vi "Main 2.0.vi"() -> ()   [LabVIEW 2019]
uses:
  Controls/Tab Button.ctl
  Controls/Main-state.ctl
  Controls/FGV States.ctl
  Controls/eFGV States.ctl
  <vilib>/Utility/miscctls.llb/LVRectTypeDef.ctl
  Controls/UDP - Command.ctl
  Controls/UDP - Event.ctl
  Controls/UDP - Status.ctl
  Controls/Global - Data UDP.vi
  <vilib>/httpClient/POSTBuffer.vi
  Controls/Global - IP Address.vi
  Controls/Global - Handle.vi
  Controls/Global - Handle V1.vi
  Controls/Global - Device.vi
  Controls/Global - Done.vi
  Controls/Global - Comport.vi
  Controls/Global - Unit.vi
  Controls/Global - ADC.vi
  Controls/Global - PID.vi
  Controls/Global - System.vi
  Controls/Global - Test.vi
  Controls/Global - Channel.vi
  <vilib>/httpClient/LabVIEWHTTPClient.lvlib
panel:
  out "error out":errorcluster
  out "Close Panel":T1
  in  "View 2":enum16{""}(ring) caption="Enum 3"
  in  "View":enum16{"VIEW", "Explorer", "Event Logs"}(ring) caption="Enum 3"
  in  "Instrument & Controls":T2(ring) caption="Enum 3"
  in  "Maintain Record":T3(ring) caption="Enum 3"
  in  "File":T4(ring) caption="Enum 3"
  in  "Path":path
  in  "Exit":bool
  in  "Data-Saturation":bool
  in  "Test Run1":bool
  in  "Next":bool
  in  "Previous":bool
  in  "Tab Array":T5
  in  "EventSwitch":bool
  out "Event":string caption="Event ^"
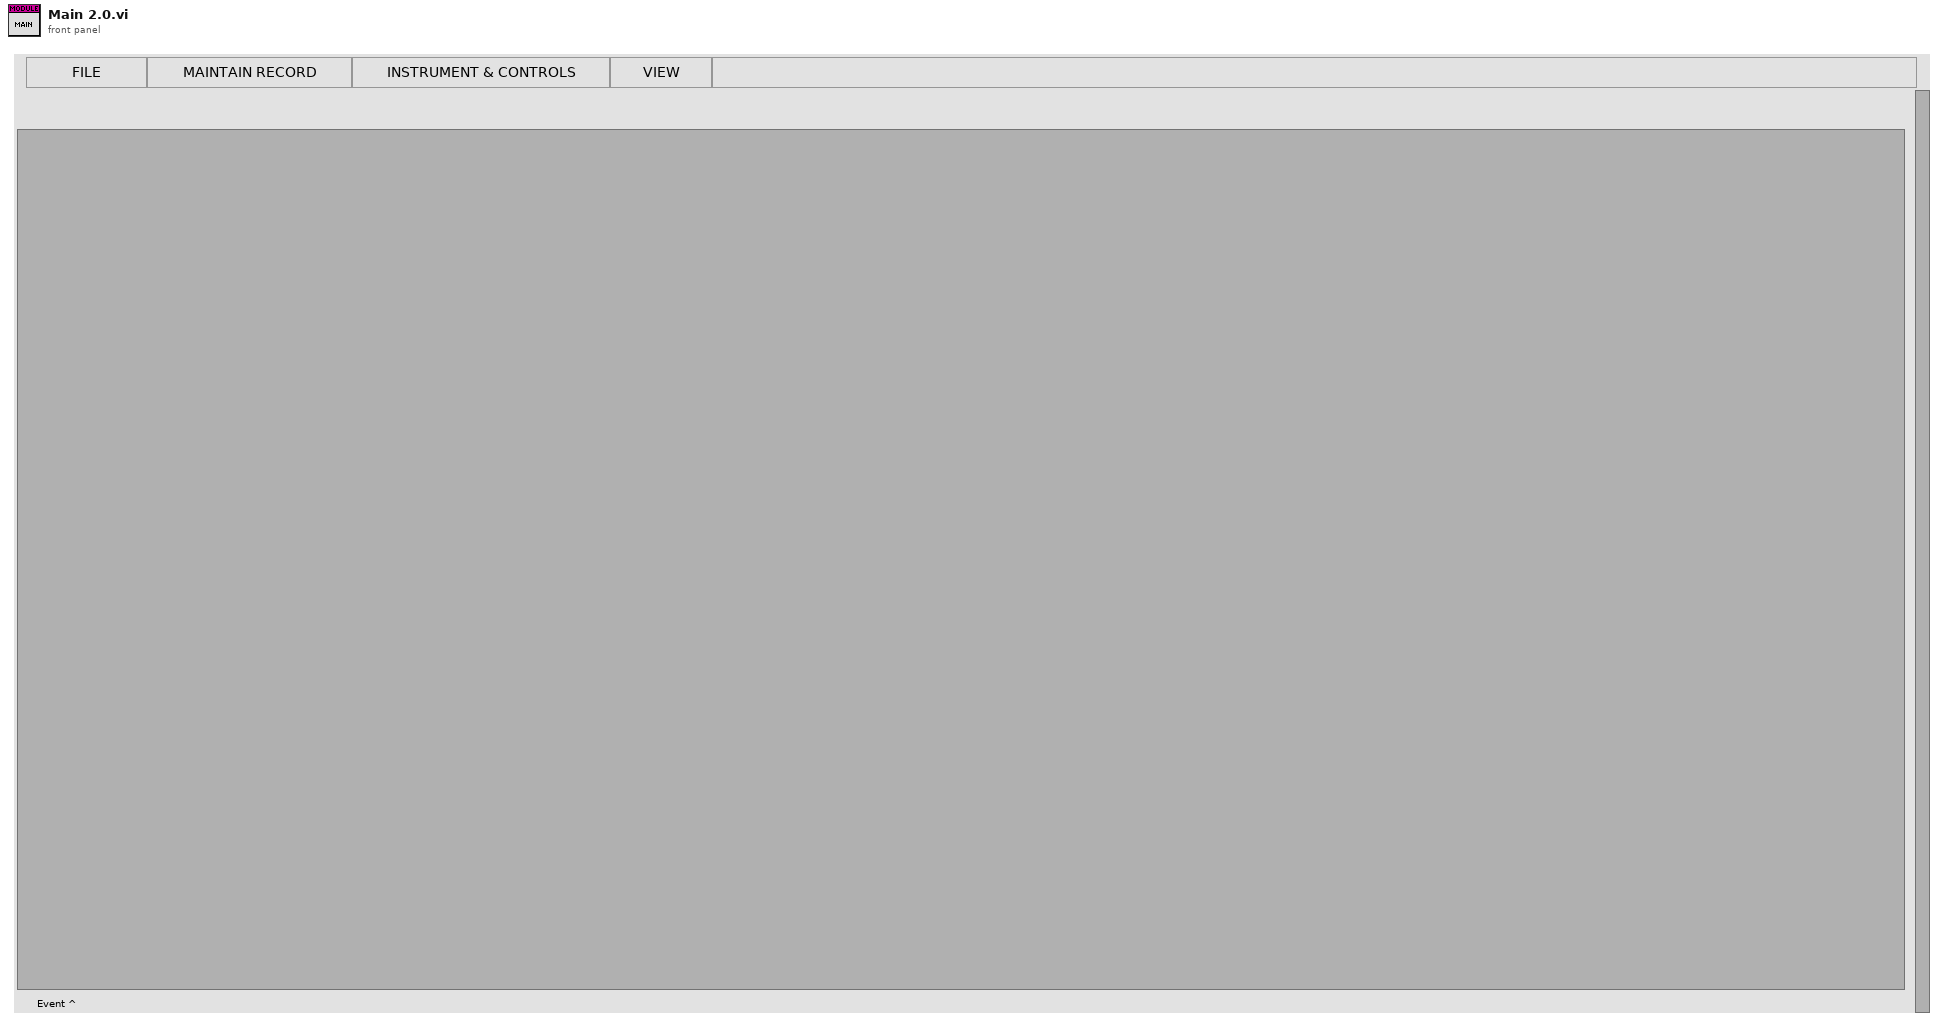
[diagram p1: front panel]
types:
  T1 = cluster{"String":string, "Cancel Button":bool, "OK Button":bool, "Bg":bool, "RunTest":refnum<vi>, "fileid":string, "Stop":bool, "Run":bool, "Status":string}
  T2 = enum16{"INSTRUMENT & CONTROLS", "Machines", "Stations", "Manual Control"}
  T3 = enum16{"MAINTAIN RECORD", "Test Plan", "Job Record"}
  T4 = enum16{"FILE", "New Test", "Export Data", "Activate License", "Emergency Stop"}
  T5 = typedef "Tab Button.ctl" = cluster{"String":string, "Cancel Button":bool, "OK Button":bool, "Bg":bool, "RunTest":refnum<vi>, "fileid":string, "Stop":bool, "Run":bool, "Status":string}[]
  T6 = enum32{"Invalid", "Standard", "Closed", "Hidden", "Minimized", "Maximized"}
  T7 = typedef "FGV States.ctl" = enum16{"Read", "Write"}
  T8 = typedef "Main-state.ctl" = enum16{"Init", "Run modules", "Idle", "Change page", "Manual Control", "NewTest", "sidepanel", "Event", "Emergency", "Exit"}
  T9 = enum32{"invalid app kind", "Development System", "Run Time System", "Student Edition", "Embedded LabVIEW", "Evaluation", "Custom"}
  T10 = cluster{"Module Ref":refnum<vi>[], "Side Name":string, "pin":bool, "FileId":string}
  T11 = typedef "eFGV States.ctl" = enum16{"Init", "Read", "Write", "Exit"}
  T12 = enum16{"New Test", "Test Plan", "Job Record", "Instrument", "Machine", "Station", "Machine Control"}
  T13 = typedef "LVRectTypeDef.ctl" = cluster{"Left":i16, "Top":i16, "Right":i16, "Bottom":i16}
  T14 = typedef "UDP - Command.ctl" = enum16{"Stop", "Jog Up", "Jog Down", "Ramp Up", "Ramp Down", "PID Target", "PID Ramp", "Disp Run", "Read Ch Data", "Zero Channel", "Zero Disp", "Read Sensor", "Write Sensor", "Read ADC", "Write ADC", "Read PID", "Write PID", "Read Test", "Write Test", "Read System", "Write System", "Read Datalog", "Read Datalog Sensor"}
  T15 = enum16{"open", "replace", "create", "open or create", "replace or create", "replace or create with confirmation"}
  T16 = cluster{"String":string, "Cancel Button":bool, "OK Button":bool, "Bg":bool, "RunTest":refnum<vi>, "fileid":string, "Stop":bool, "Run":bool, "Status":string}[]
  T17 = typedef "LabVIEWHTTPClient.lvlib/ClientHandle.ctl" = refnum<k1>
  T18 = cluster{"IP Address":string, "port":string, "UDP ref":refnum<k16>}[]
  T19 = typedef "UDP - Event.ctl" = u16
  T20 = typedef "UDP - Status.ctl" = u16
  T21 = cluster{"Channels":cluster{"Ch1":sgl, "Ch2":sgl, "Ch3":sgl, "Ch4":sgl, "Ch5":sgl, "Ch6":sgl, "Ch7":sgl, "Ch8":sgl, "Ch9":sgl, "Ch10":sgl, "Ch11":sgl, "Ch12":sgl, "Ch13":sgl, "Ch14":sgl, "Ch15":sgl, "Ch16":sgl}, "Event":T19, "Status":T20, string}[]
  T22 = cluster{"Ch1":sgl, "Ch2":sgl, "Ch3":sgl, "Ch4":sgl, "Ch5":sgl, "Ch6":sgl, "Ch7":sgl, "Ch8":sgl, "Ch9":sgl, "Ch10":sgl, "Ch11":sgl, "Ch12":sgl, "Ch13":sgl, "Ch14":sgl, "Ch15":sgl, "Ch16":sgl}
  T23 = cluster{"Target Load":sgl, "Target Disp":sgl, "Rate":sgl, "Speed":sgl}[]
  T24 = cluster{"Out Type":u8, "Inverse":u8, "Monitor":u8, "Reserve":u8, "ACC Time":u32, "Pulse Rev":u32, "Stroke":u32, "Auto Off":u32, "Gear Ratio":sgl, "Pitch":sgl, "Max Speed":u32, "Jog Speed":u32, "Disp Coff":sgl, "Max Load":u32}[]
  T25 = cluster{"SP":sgl, "PV":sgl, "kP":sgl, "kI":sgl, "kD":sgl, "FF":sgl, "Err Band":sgl, "Max":i32, "Min":i32, "Ts":u32, "Out":i32, "Mode":u8}[]
  T26 = cluster{"Active Ch":u8[], "Filter Type":u8, "Post Filter":u8[], "Gain":u8[], "FS":u16, "IntOC":u8, "IntFC":u8, "SysOC":u8, "Cofficient":dbl[], "K":dbl[], "Max":i32}[]
  T27 = cluster{"Name":string[], "Unit":string[], "Decimal Point":u8[], "Ch Log":u8[], "H Alarm":u8[], "L Alarm":u8[], "H Limit":sgl[], "L Limit":sgl[], "Filter":u8[], "Gain":u8[], "Calib Type":u32[]}[]
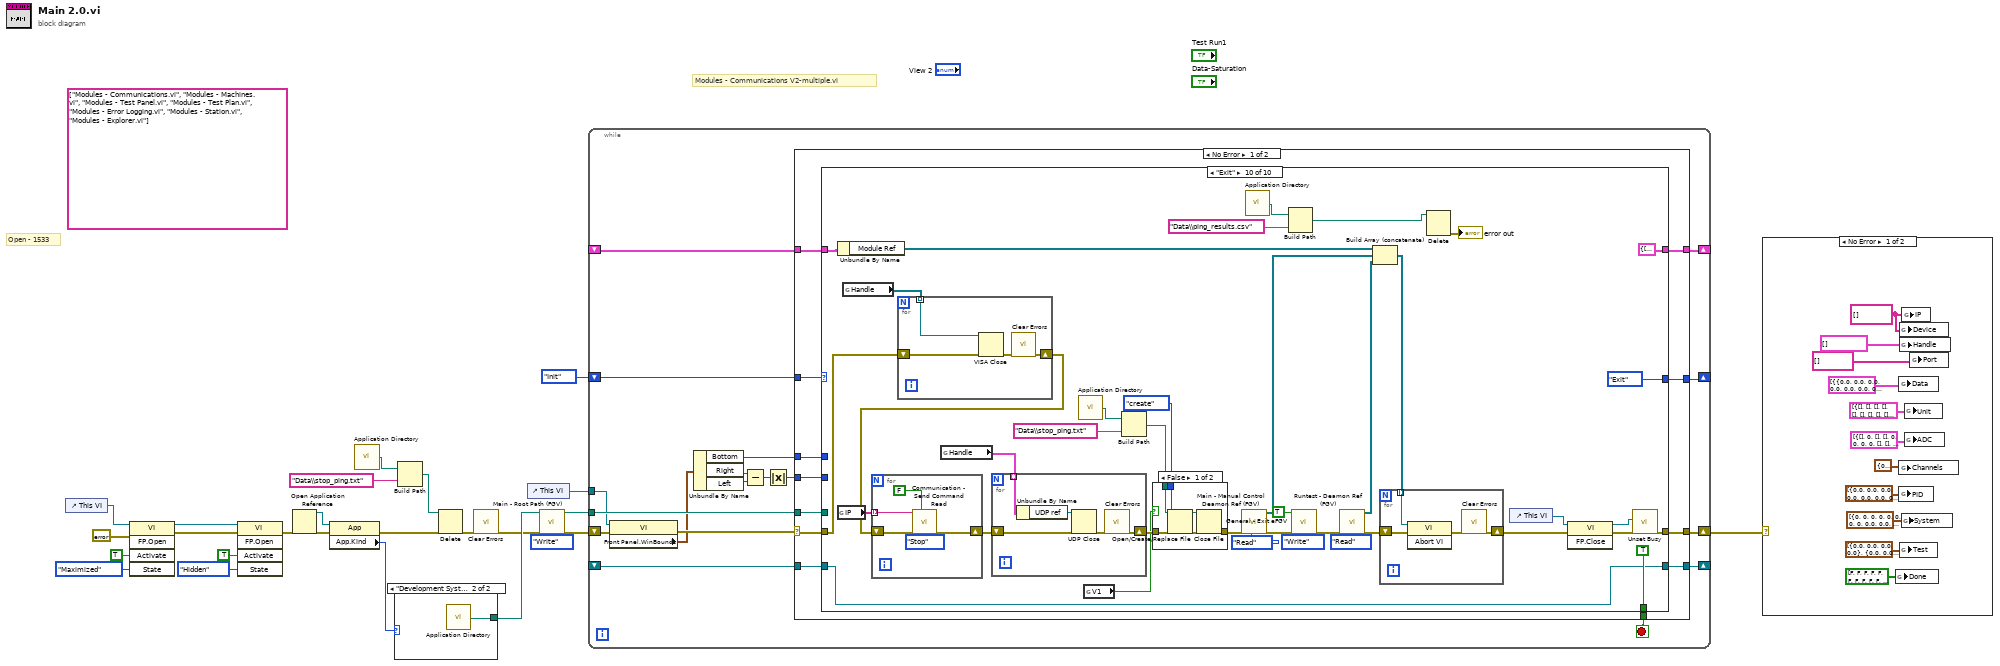
[diagram p0: block diagram]
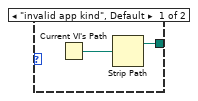
[diagram p2: hidden frame]
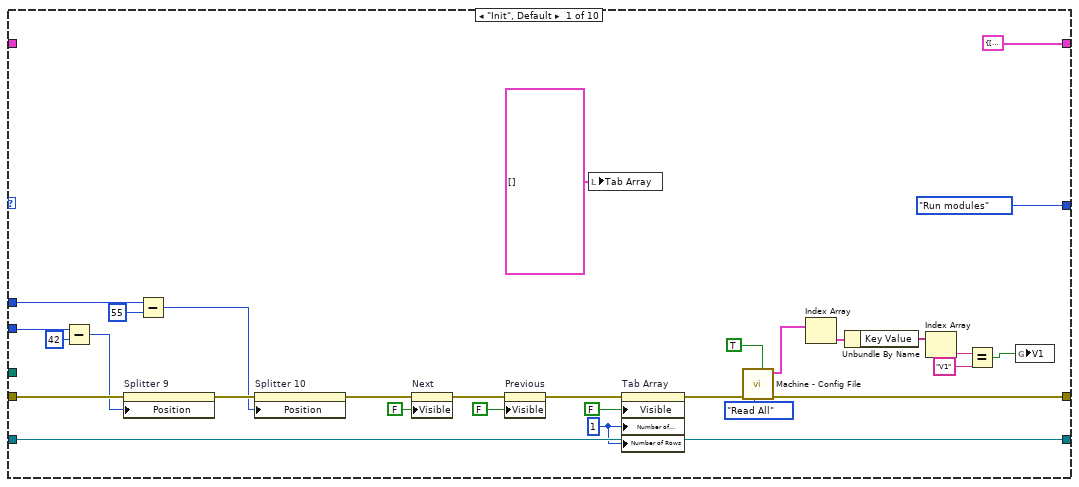
[diagram p3: hidden frame]
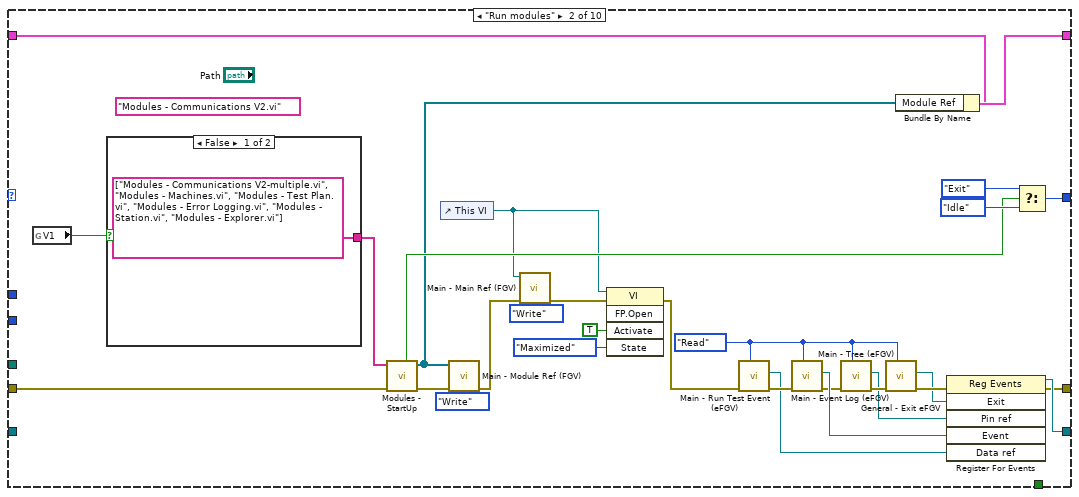
[diagram p4: hidden frame]
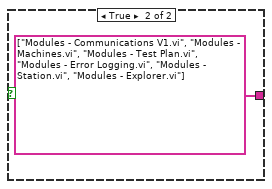
[diagram p5: hidden frame]
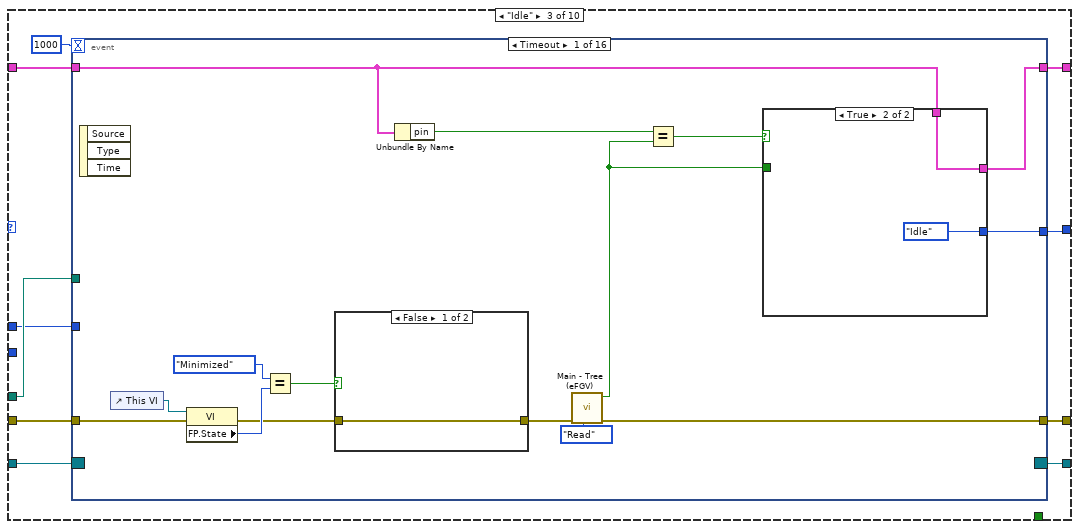
[diagram p6: hidden frame]
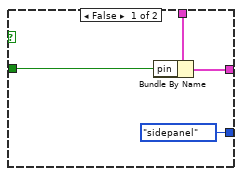
[diagram p7: hidden frame]
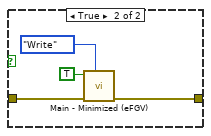
[diagram p8: hidden frame]
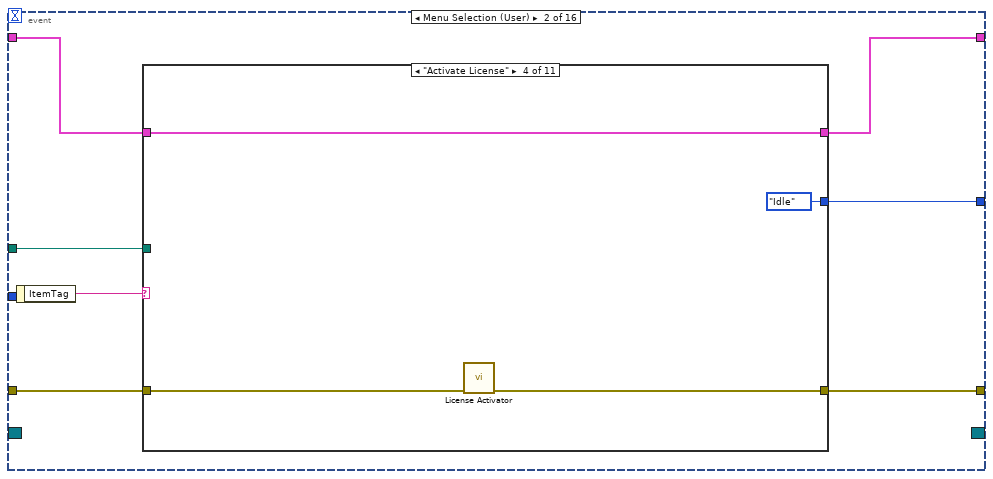
[diagram p9: hidden frame]
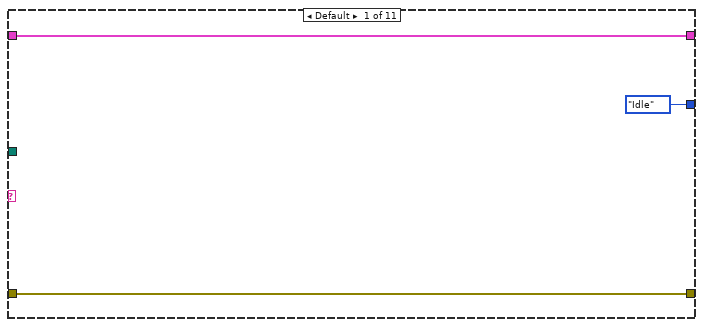
[diagram p10: hidden frame]
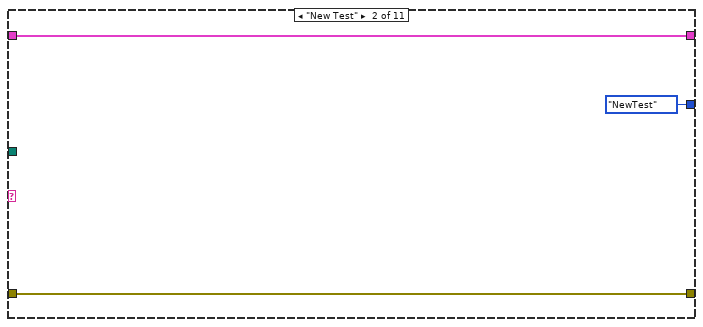
[diagram p11: hidden frame]
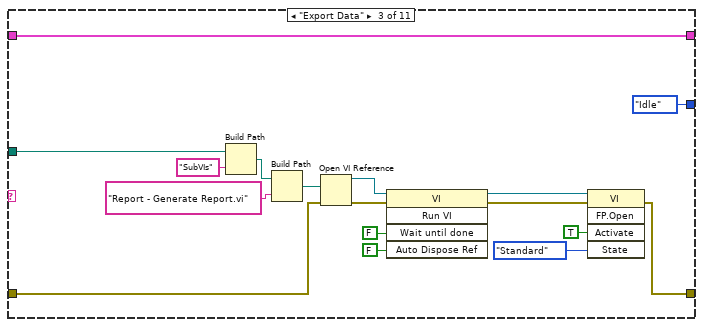
[diagram p12: hidden frame]
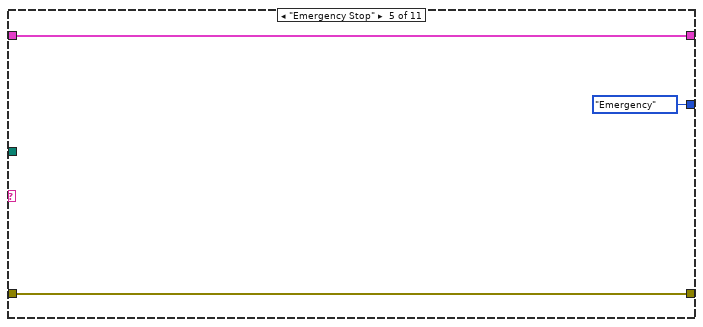
[diagram p13: hidden frame]
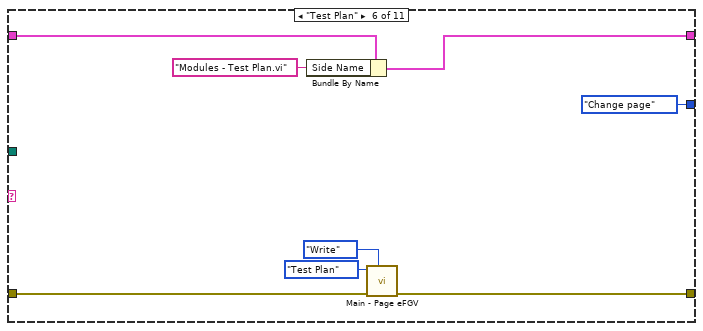
[diagram p14: hidden frame]
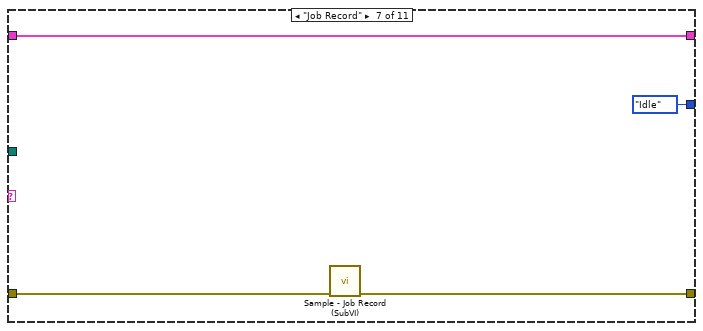
[diagram p15: hidden frame]
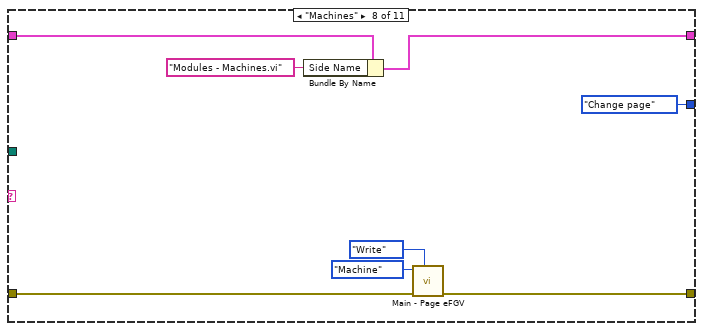
[diagram p16: hidden frame]
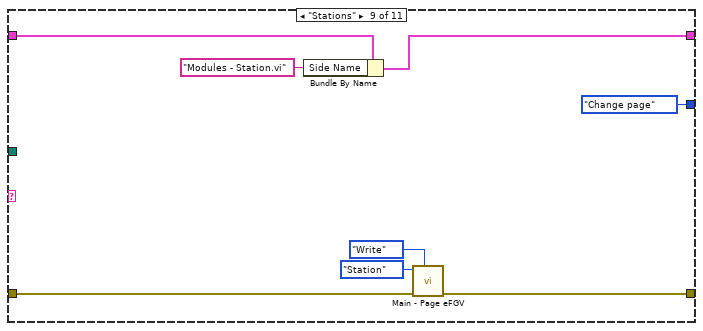
[diagram p17: hidden frame]
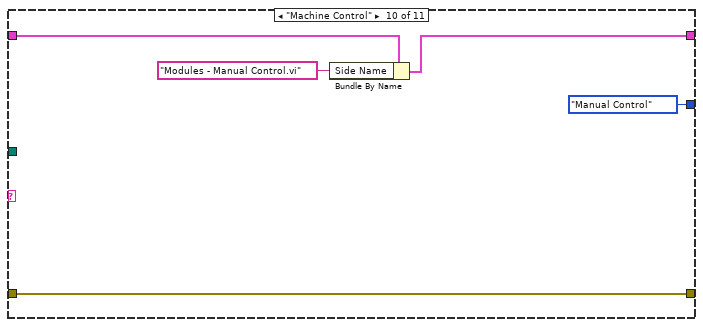
[diagram p18: hidden frame]
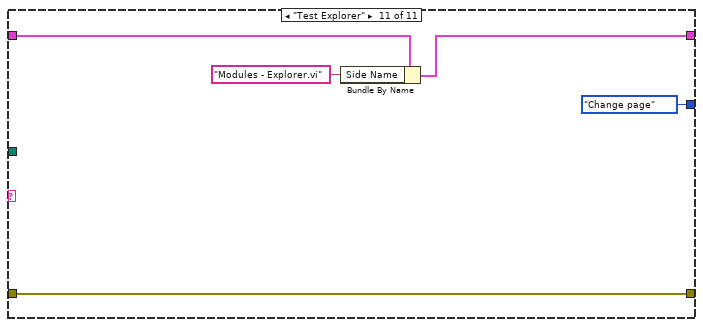
[diagram p19: hidden frame]
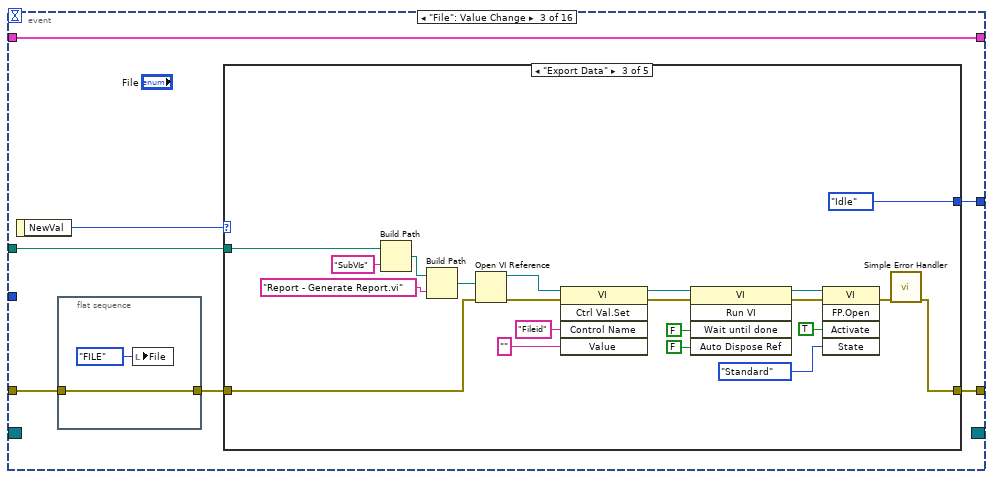
[diagram p20: hidden frame]
diagram:
  (unwired) string[] ["Modules - Communications.vi", "Modules - Machines.vi", "Modules - Test Panel.vi", "Modules - Test Plan.vi", "Modules - Error Logging.vi", "Modules - Station.vi", "Modules - Explorer.vi"]
  # "Modules - Communications V2-multiple.vi"
  # "Open - 1533"
  n1 = control-ref of="This VI"() -> (w16:refnum<vi>)
  n2 = invoke class="VI" method="FP.Open"(reference=w16, error in=errorcluster {"status"=FALSE, "code"=0, "source"=""} ("error in (no error)"), "Activate"=TRUE ("Activate?"), "State"=T6."Maximized") -> (reference out=w7:refnum<vi>, error out=w9:errorcluster)  [unwired: 1 in, 3 out]
  n3 = invoke class="VI" method="FP.Open"(reference=w7, error in=w9, "Activate"=TRUE ("Activate?"), "State"=T6."Hidden") -> (error out=w8:errorcluster)  [unwired: 1 in, 4 out]
  n4 = Open Application Reference(8:w8) -> (0:w15:errorcluster, 3:w14:refnum<vi>)  [unwired: 3 in]
  n5 = property class="App"(reference=w14, error in=w15) -> (error out=w3:errorcluster, "App.Kind"=w13:T9)  [unwired: 1 out]
  n6 = call <vilib>:"Application Directory.vi"() -> ("Application Directory"=w6:path)
  n7 = case shown="\"Development System\"" w13 {
    tunnel: [w26 w28] -> w25
    frame "invalid app kind", Default {
      n8 = Current VI's Path() -> (path=w27:path)
      n9 = Strip Path(path=w27) -> (stripped path=w26:path)  [unwired: 1 out]
    }
    frame "Development System" {
      n10 = call <vilib>:"Application Directory.vi"() -> ("Application Directory"=w28:path)
    }
  }
  n11 = Build Path(base path=w6, name or relative path="Data\\stop_ping.txt") -> (appended path=w4:path)
  n12 = Delete(path (use dialog)=w4, error in=w3) -> (error out=w2:errorcluster)  [unwired: 3 in, 2 out]
  n13 = call <vilib>:"Clear Errors.vi"("error in (no error)"=w2) -> ("error out"=w1:errorcluster)  [unwired: 5 in, 1 out]
  n14 = control-ref of="This VI"() -> (w19:refnum<vi>)
  n15 = call "Main - Root Path (FGV).vi"("Action"=FGV_States."Write", "error in"=w1, "Path in"=w25) -> ("error out"=w22:errorcluster, "Path out"=w20:path)  [unwired: 7 in]
  n16 = while {
    shift-right: [w44] -> _
    shift-left: Main-state."Init" -> [w46]
    shift-right: [w45] -> w24
    shift-left: w22 -> [w37]
    shift-right: [w42] -> _
    shift-left: _ -> [w41]
    shift-right: [w40] -> _
    shift-left: _ -> [w39]
    tunnel: w20 -> [w38]
    tunnel: w19 -> [w36]
    stop <- w43 stop-if-true
    n17 = property class="VI"(reference=w36, error in=w37) -> (error out=w35:errorcluster, "Front Panel.WinBounds"=w34:T13)  [unwired: 1 out]
    n18 = Unbundle By Name(w34) -> ("Bottom"=w29:i16, "Right"=w32:i16, "Left"=w33:i16)
    n19 = Subtract(x=w32, y=w33) -> (x-y=w31:i16)
    n20 = Absolute Value(x=w31) -> (abs(x)=w30:i16)
    n21 = case shown="No Error" w35 {
      selector: w35 -> [w57 w891]
      tunnel: w46 -> [w58 _]
      tunnel: [w56 w888] -> w45
      tunnel: [w55 Main-state."Idle"] -> w44
      tunnel: [w54 _] -> w43
      tunnel: [w53 w890] -> w42
      tunnel: w41 -> [w52 w890]
      tunnel: [w51 w886] -> w40
      tunnel: w39 -> [w50 w886]
      tunnel: w38 -> [w49 _]
      tunnel: w30 -> [w48 _]
      tunnel: w29 -> [w47 _]
      frame No Error {
        n22 = case shown="\"Exit\"" w58 {
          tunnel: w57 -> [w67 w115 w128 w592 w630 w675 w695 w741 w799 w824]
          tunnel: [w76 w95 w129 w595 w635 w674 w698 w736 w798 w848] -> w56
          tunnel: [Main-state."Run modules" w110 w125 Main-state."Idle" Main-state."Idle" Main-state."Idle" Main-state."Idle" Main-state."Idle" Main-state."Idle" Main-state."Exit"] -> w55
          tunnel: [_ _ _ _ _ _ _ _ _ TRUE] -> w54
          tunnel: [T10 {"Module Ref"=[], "Side Name"="", "pin"=FALSE, "FileId"=""} w117 w126 w594 w638 w687 w697 w740 w805 T10 {"Module Ref"=[], "Side Name"="", "pin"=FALSE, "FileId"=""}] -> w53
          tunnel: w52 -> [_ w94 w127 w594 w638 w687 w697 w740 w805 w856]
          tunnel: [w86 w103 w122 w588 w639 w688 w700 w745 w806 w846] -> w51
          tunnel: w50 -> [w86 _ w123 w588 w639 w688 w700 w745 w806 w846]
          tunnel: w49 -> [_ _ w121 _ w626 w682 _ _ _ _]
          tunnel: w48 -> [w64 _ _ _ _ w671 w689 _ _ _]
          tunnel: w47 -> [w61 _ w120 _ _ _ _ _ _ _]
          frame "Init", Default {
            w80 = u32 1 ("Number of Columns")
            n23 = Subtract(x=w64, y=i16 42) -> (x-y=w65:i16)
            n24 = property on="Splitter 9" class="Splitter"(error in=w67, "Position"=w65) -> (error out=w63:errorcluster)  [unwired: 1 in, 1 out]
            n25 = Subtract(x=w61, y=i16 55) -> (x-y=w60:i16)
            n26 = property on="Splitter 10" class="Splitter"(error in=w63, "Position"=w60) -> (error out=w62:errorcluster)  [unwired: 1 in, 1 out]
            n27 = property on="Next" class="Bool"(error in=w62, "Visible"=FALSE) -> (error out=w83:errorcluster)  [unwired: 1 in, 1 out]
            n28 = property on="Previous" class="Bool"(error in=w83, "Visible"=FALSE) -> (error out=w82:errorcluster)  [unwired: 1 in, 1 out]
            n29 = local write "Tab Array"(T5 [] ("Array")) -> ()
            n30 = property on="Tab Array" class="Arr"(error in=w82, "Visible"=FALSE, "Number of Columns"=w80, "Number of Rows"=w80) -> (error out=w77:errorcluster)  [unwired: 1 in, 1 out]
            n31 = call "Machine - Config File.vi"("Setting"=TRUE, "Action"=enum16{"Write", "Read", "Read All", "Remove"}."Read All", "error in (no error)"=w77) -> ("error out"=w76:errorcluster, "Value Out"=w72:cluster{"IP/SN":string, "Key Value":string[]}[])  [unwired: 7 in]
            n32 = Index Array(array=w72) -> (element=w74:cluster{"IP/SN":string, "Key Value":string[]})  [unwired: 1 in]
            n33 = Unbundle By Name(w74) -> ("Key Value"=w73:string[])
            n34 = Index Array(array=w73) -> (element=w70:string)  [unwired: 1 in]
            n35 = Equal?(x=w70, y="V1") -> (x = y?=w68:bool)
            n36 = global write "Global - Data UDP.vi" "V1"(w68) -> ()
          }
          frame "Run modules" {
            (unwired) "Modules - Communications V2.vi"
            w90 = eFGV_States."Read" ("Action")
            n37 = global read "Global - Data UDP.vi" "V1"() -> (w93:bool)
            n38 = case shown="False" w93 {
              tunnel: [string[] ["Modules - Communications V2-multiple.vi", "Modules - Machines.vi", "Modules - Test Plan.vi", "Modules - Error Logging.vi", "Modules - Station.vi", "Modules - Explorer.vi"] string[] ["Modules - Communications V1.vi", "Modules - Machines.vi", "Modules - Test Plan.vi", "Modules - Error Logging.vi", "Modules - Station.vi", "Modules - Explorer.vi"]] -> w116
              frame False {
              }
              frame True {
              }
            }
            n39 = call "Modules - StartUp.vi"("Error In"=w115, "List of Modules"=w116) -> ("Error Out"=w107:errorcluster, "Module Ref"=w106:refnum<vi>[], "Force Exit"=w109:bool)  [unwired: 7 in]
            n40 = control-ref of="This VI"() -> (w100:refnum<vi>)
            n41 = call "Main - Module Ref (FGV).vi"("Action"=FGV_States."Write", "error in"=w107, "Ref in"=w106) -> ("error out"=w102:errorcluster)  [unwired: 7 in, 1 out]
            n42 = call "Main - Main Ref (FGV).vi"("Action"=FGV_States."Write", "error in"=w102, "This VI"=w100) -> ("error out"=w101:errorcluster)  [unwired: 7 in, 1 out]
            n43 = invoke class="VI" method="FP.Open"(reference=w100, error in=w101, "Activate"=TRUE ("Activate?"), "State"=T6."Maximized") -> (error out=w97:errorcluster)  [unwired: 1 in, 4 out]
            n44 = call "Main - Run Test Event (eFGV).vi"("Action"=w90, "error in"=w97) -> ("error out"=w96:errorcluster, "Data ref"=w88:refnum<user-event>)  [unwired: 7 in, 1 out]
            n45 = call "Main - Event Log (eFGV).vi"("Action"=w90, "error in"=w96) -> ("error out"=w92:errorcluster, "Event"=w98:refnum<user-event>)  [unwired: 6 in, 2 out]
            n46 = call "Main - Tree (eFGV).vi"("Action"=w90, "error in"=w92) -> ("error out"=w91:errorcluster, "Pin ref"=w89:refnum<user-event>)  [unwired: 7 in, 1 out]
            n47 = call "General - Exit eFGV.vi"("eFGV States"=w90, "error in (no error)"=w91) -> ("error out"=w105:errorcluster, "Exit"=w104:refnum<user-event>)  [unwired: 7 in, 1 out]
            n48 = Bundle By Name(cluster=w94, "Module Ref"=w106) -> (w117:T10)
            n49 = register-events(error in=w105, w104, w89, w98, w88) -> (reference out=w103:refnum<event-registration>, error out=w95:errorcluster)  [unwired: 1 in]
            n50 = Select(t=Main-state."Exit", s=w109, f=Main-state."Idle") -> (s? t:f=w110:T8)
          }
          frame "Idle" {
            n51 = event shown="[0] Timeout" {
              selector: w123 -> [_ _ _ _ _ _ _ _ _ _ _ _ _ _ _ _]
              dyn-events: [_ _ _ _ _ _ _ _ _ _ _ _ _ _ _ _] -> w122
              timeout: 1000 -> [_ _ _ _ _ _ _ _ _ _ _ _ _ _ _ _]
              tunnel: [w136 w162 w234 w270 w295 w328 w364 w368 w374 w377 w380 w392 w413 w439 w516 w573] -> w129
              tunnel: w128 -> [w142 w161 w233 w275 w299 w333 w364 w368 w374 w377 w381 w391 w412 w441 w515 w579]
              tunnel: w127 -> [w131 w158 w237 w272 w296 w331 w363 w366 w371 w375 w383 w403 w424 w437 w523 w585]
              tunnel: [w132 w157 w237 w273 w297 w332 w363 w367 w372 w375 w383 w403 w424 w438 w523 w585] -> w126
              tunnel: [w144 w159 w235 w274 w298 w330 Main-state."Exit" Main-state."Event" Main-state."sidepanel" Main-state."Exit" w384 Main-state."Idle" Main-state."Idle" w435 Main-state."Idle" Main-state."Idle"] -> w125
              tunnel: w121 -> [_ w156 w231 _ _ w327 _ _ _ _ _ _ _ _ _ _]
              tunnel: w120 -> [_ _ _ _ _ _ _ _ _ _ _ _ _ _ _ w583]
              event Timeout {
                n52 = event-data() -> ()  [unwired: 1 in, 3 out]
                n53 = control-ref of="This VI"() -> (w143:refnum<vi>)
                n54 = property class="VI"(reference=w143, error in=w142) -> (error out=w138:errorcluster, "FP.State"=w140:T6)  [unwired: 1 out]
                n55 = Equal?(x=T6."Minimized" ("Front Panel Window:State"), y=w140) -> (x = y?=w139:bool)
                n56 = case shown="False" w139 {
                  tunnel: [w151 w154] -> w137
                  tunnel: w138 -> [w151 w155]
                  frame False {
                  }
                  frame True {
                    n57 = call "Main - Minimized (eFGV).vi"("Action"=eFGV_States."Write", "error in"=w155, "Minimized In"=TRUE) -> ("error out"=w154:errorcluster)  [unwired: 6 in, 2 out]
                  }
                }
                n58 = Unbundle By Name(w131) -> ("pin"=w134:bool)
                n59 = call "Main - Tree (eFGV).vi"("Action"=eFGV_States."Read", "error in"=w137) -> ("error out"=w136:errorcluster, "Pin out"=w130:bool)  [unwired: 7 in, 1 out]
                n60 = Equal?(x=w134, y=w130) -> (x = y?=w133:bool)
                n61 = case shown="True" w133 {
                  tunnel: [Main-state."sidepanel" Main-state."Idle"] -> w144
                  tunnel: w131 -> [w147 w149]
                  tunnel: [w146 w149] -> w132
                  tunnel: w130 -> [w145 _]
                  frame False {
                    n62 = Bundle By Name(cluster=w147, "pin"=w145) -> (w146:T10)
                  }
                  frame True {
                  }
                }
              }
              event Menu Selection (User) {
                n63 = event-data() -> ("ItemTag"=w160:string)  [unwired: 1 in]
                n64 = case shown="\"Activate License\"" w160 {
                  tunnel: [w165 w168 w170 w187 w191 w196 w202 w208 w216 w225 w230] -> w162
                  tunnel: w161 -> [w165 w168 w171 w186 w191 w195 w201 w207 w215 w225 w230]
                  tunnel: [Main-state."Idle" Main-state."NewTest" Main-state."Idle" Main-state."Idle" Main-state."Emergency" Main-state."Change page" Main-state."Idle" Main-state."Change page" Main-state."Change page" Main-state."Manual Control" Main-state."Change page"] -> w159
                  tunnel: [w163 w166 w184 w189 w190 w194 w203 w206 w214 w223 w227] -> w157
                  tunnel: w158 -> [w163 w166 w184 w189 w190 w193 w203 w205 w213 w222 w226]
                  tunnel: w156 -> [_ _ w169 _ _ _ _ _ _ _ _]
                  frame Default {
                  }
                  frame "New Test" {
                  }
                  frame "Export Data" {
                    n65 = Build Path(base path=w169, name or relative path="SubVIs") -> (appended path=w182:path)
                    n66 = Build Path(base path=w182, name or relative path="Report - Generate Report.vi") -> (appended path=w183:path)
                    n67 = Open VI Reference(vi path=w183, error in (no error)=w171) -> (vi reference=w172:refnum<vi>, error out=w181:errorcluster)  [unwired: 4 in]
                    n68 = invoke class="VI" method="Run VI"(reference=w172, error in=w181, "Wait until done"=FALSE ("Wait Until Done"), "Auto Dispose Ref"=FALSE ("Auto Dispose Reference")) -> (reference out=w180:refnum<vi>, error out=w179:errorcluster)  [unwired: 1 in, 3 out]
                    n69 = invoke class="VI" method="FP.Open"(reference=w180, error in=w179, "Activate"=TRUE ("Activate?"), "State"=T6."Standard") -> (error out=w170:errorcluster)  [unwired: 1 in, 4 out]
                  }
                  frame "Activate License" {
                    n70 = call "License Activator.vi"("error constant"=w186) -> ("error out"=w187:errorcluster)  [unwired: 10 in]
                  }
                  frame "Emergency Stop" {
                  }
                  frame "Test Plan" {
                    n71 = Bundle By Name(cluster=w193, "Side Name"="Modules - Test Plan.vi") -> (w194:T10)
                    n72 = call "Main - Page eFGV.vi"("eFGV States"=eFGV_States."Write", "error in (no error)"=w195, "Page In"=T12."Test Plan") -> ("error out"=w196:errorcluster)  [unwired: 6 in, 2 out]
                  }
                  frame "Job Record" {
                    n73 = call "Sample - Job Record (SubVI).vi"("error in"=w201) -> ("error out"=w202:errorcluster)  [unwired: 10 in]
                  }
                  frame "Machines" {
                    n74 = Bundle By Name(cluster=w205, "Side Name"="Modules - Machines.vi") -> (w206:T10)
                    n75 = call "Main - Page eFGV.vi"("eFGV States"=eFGV_States."Write", "error in (no error)"=w207, "Page In"=T12."Machine") -> ("error out"=w208:errorcluster)  [unwired: 6 in, 2 out]
                  }
                  frame "Stations" {
                    n76 = Bundle By Name(cluster=w213, "Side Name"="Modules - Station.vi") -> (w214:T10)
                    n77 = call "Main - Page eFGV.vi"("eFGV States"=eFGV_States."Write", "error in (no error)"=w215, "Page In"=T12."Station") -> ("error out"=w216:errorcluster)  [unwired: 6 in, 2 out]
                  }
                  frame "Machine Control" {
                    n78 = Bundle By Name(cluster=w222, "Side Name"="Modules - Manual Control.vi") -> (w223:T10)
                  }
                  frame "Test Explorer" {
                    n79 = Bundle By Name(cluster=w226, "Side Name"="Modules - Explorer.vi") -> (w227:T10)
                  }
                }
              }
              event "File": Value Change {
                n80 = event-data() -> ("NewVal"=w236:T4)  [unwired: 1 in]
                n81 = flat-sequence {
                  tunnel: [w239] -> w232
                  tunnel: w233 -> [w239]
                  frame #0 {
                    n82 = local write "File"(T4."FILE" ("File")) -> ()
                  }
                }
                n83 = case shown="\"Export Data\"" w236 {
                  tunnel: [Main-state."Idle" Main-state."NewTest" Main-state."Idle" Main-state."Idle" Main-state."Emergency"] -> w235
                  tunnel: w232 -> [w240 w242 w263 w266 w268]
                  tunnel: [w240 w242 w244 w265 w268] -> w234
                  tunnel: w231 -> [_ _ w262 _ _]
                  frame "FILE", Default {
                  }
                  frame "New Test" {
                  }
                  frame "Export Data" {
                    n84 = Build Path(base path=w262, name or relative path="SubVIs") -> (appended path=w260:path)
                    n85 = Build Path(base path=w260, name or relative path="Report - Generate Report.vi") -> (appended path=w261:path)
                    n86 = Open VI Reference(vi path=w261, error in (no error)=w263) -> (vi reference=w246:refnum<vi>, error out=w249:errorcluster)  [unwired: 4 in]
                    n87 = invoke class="VI" method="Ctrl Val.Set"(reference=w246, error in=w249, "Control Name"="Fileid", "Value"="" ("Control Name")) -> (reference out=w247:refnum<vi>, error out=w248:errorcluster)  [unwired: 1 in, 3 out]
                    n88 = invoke class="VI" method="Run VI"(reference=w247, error in=w248, "Wait until done"=FALSE ("Wait Until Done"), "Auto Dispose Ref"=FALSE ("Auto Dispose Reference")) -> (reference out=w259:refnum<vi>, error out=w258:errorcluster)  [unwired: 1 in, 3 out]
                    n89 = invoke class="VI" method="FP.Open"(reference=w259, error in=w258, "Activate"=TRUE ("Activate?"), "State"=T6."Standard") -> (error out=w245:errorcluster)  [unwired: 1 in, 4 out]
                    n90 = call <vilib>:"Simple Error Handler.vi"("error in (no error)"=w245) -> ("error out"=w244:errorcluster)  [unwired: 4 in, 4 out]
                  }
                  frame "Activate License" {
                    n91 = call "License Activator.vi"("error constant"=w266) -> ("error out"=w265:errorcluster)  [unwired: 10 in]
                  }
                  frame "Emergency Stop" {
                  }
                }
              }
              event "Maintain Record": Value Change {
                n92 = event-data() -> ("NewVal"=w276:T3)  [unwired: 1 in]
                n93 = case shown="\"MAINTAIN RECORD\", Default" w276 {
                  tunnel: w275 -> [w281 w286 w291]
                  tunnel: [w281 w285 w292] -> w271
                  tunnel: [Main-state."Idle" Main-state."Change page" Main-state."Idle"] -> w274
                  tunnel: w272 -> [w280 w283 w293]
                  tunnel: [w280 w282 w293] -> w273
                  frame "MAINTAIN RECORD", Default {
                  }
                  frame "Test Plan" {
                    n94 = Bundle By Name(cluster=w283, "Side Name"="Modules - Test Plan.vi") -> (w282:T10)
                    n95 = call "Main - Page eFGV.vi"("eFGV States"=eFGV_States."Write", "error in (no error)"=w286, "Page In"=T12."Test Plan") -> ("error out"=w285:errorcluster)  [unwired: 6 in, 2 out]
                  }
                  frame "Job Record" {
                    n96 = call "Sample - Job Record (SubVI).vi"("error in"=w291) -> ("error out"=w292:errorcluster)  [unwired: 10 in]
                  }
                }
                n97 = flat-sequence {
                  tunnel: [w278] -> w270
                  tunnel: w271 -> [w278]
                  frame #0 {
                    n98 = local write "Maintain Record"(0) -> ()
                  }
                }
              }
              event "Instrument & Controls": Value Change {
                n99 = event-data() -> ("NewVal"=w300:T2)  [unwired: 1 in]
                n100 = case shown="\"Manual Control\"" w300 {
                  tunnel: w299 -> [w305 w310 w318 w325]
                  tunnel: [w305 w309 w317 w325] -> w294
                  tunnel: [Main-state."Idle" Main-state."Change page" Main-state."Change page" Main-state."Manual Control"] -> w298
                  tunnel: w296 -> [w304 w307 w315 w323]
                  tunnel: [w304 w306 w314 w322] -> w297
                  frame "INSTRUMENT & CONTROLS", Default {
                  }
                  frame "Machines" {
                    n101 = Bundle By Name(cluster=w307, "Side Name"="Modules - Machines.vi") -> (w306:T10)
                    n102 = call "Main - Page eFGV.vi"("eFGV States"=eFGV_States."Write", "error in (no error)"=w310, "Page In"=T12."Machine") -> ("error out"=w309:errorcluster)  [unwired: 6 in, 2 out]
                  }
                  frame "Stations" {
                    n103 = Bundle By Name(cluster=w315, "Side Name"="Modules - Station.vi") -> (w314:T10)
                    n104 = call "Main - Page eFGV.vi"("eFGV States"=eFGV_States."Write", "error in (no error)"=w318, "Page In"=T12."Station") -> ("error out"=w317:errorcluster)  [unwired: 6 in, 2 out]
                  }
                  frame "Manual Control" {
                    n105 = Bundle By Name(cluster=w323, "Side Name"="Modules - Manual Control.vi") -> (w322:T10)
                  }
                }
                n106 = flat-sequence {
                  tunnel: [w301] -> w295
                  tunnel: w294 -> [w301]
                  frame #0 {
                    n107 = local write "Instrument & Controls"(0) -> ()
                  }
                }
              }
              event "View": Value Change {
                n108 = event-data() -> ("NewVal"=w334:enum16{"VIEW", "Explorer", "Event Logs"})  [unwired: 1 in]
                n109 = case shown="\"Explorer\"" w334 {
                  tunnel: [w339 w344 w347] -> w329
                  tunnel: w333 -> [w339 w344 w346]
                  tunnel: w331 -> [w338 w342 w360]
                  tunnel: [w338 w341 w360] -> w332
                  tunnel: [Main-state."Idle" Main-state."Change page" Main-state."Idle"] -> w330
                  tunnel: w327 -> [_ _ w345]
                  frame "VIEW", Default {
                  }
                  frame "Explorer" {
                    n110 = Bundle By Name(cluster=w342, "Side Name"="Modules - Explorer.vi") -> (w341:T10)
                  }
                  frame "Event Logs" {
                    n111 = Build Path(base path=w345, name or relative path="SubVIs") -> (appended path=w356:path)
                    n112 = Build Path(base path=w356, name or relative path="Event - Load Event Log.vi") -> (appended path=w357:path)
                    n113 = Open VI Reference(vi path=w357, error in (no error)=w346) -> (vi reference=w359:refnum<vi>, error out=w358:errorcluster)  [unwired: 4 in]
                    n114 = invoke class="VI" method="Run VI"(reference=w359, error in=w358, "Wait until done"=FALSE ("Wait Until Done"), "Auto Dispose Ref"=FALSE ("Auto Dispose Reference")) -> (reference out=w355:refnum<vi>, error out=w354:errorcluster)  [unwired: 1 in, 3 out]
                    n115 = invoke class="VI" method="FP.Open"(reference=w355, error in=w354, "Activate"=TRUE ("Activate?"), "State"=T6."Standard") -> (error out=w347:errorcluster)  [unwired: 1 in, 4 out]
                  }
                }
                n116 = flat-sequence {
                  tunnel: [w336] -> w328
                  tunnel: w329 -> [w336]
                  frame #0 {
                    n117 = local write "View"(0) -> ()
                  }
                }
              }
              event User Event {
                n118 = event-data() -> ()  [unwired: 1 in, 5 out]
              }
              event User Event {
                n119 = event-data() -> ("fileid"=w365:string)  [unwired: 1 in]
                n120 = Bundle By Name(cluster=w366, "FileId"=w365) -> (w367:T10)
              }
              event User Event {
                n121 = event-data() -> ("Pin"=w370:bool)  [unwired: 1 in]
                n122 = Bundle By Name(cluster=w371, "pin"=w370) -> (w372:T10)
              }
              event "Exit": Value Change {
                n123 = event-data() -> ()  [unwired: 1 in, 1 out]
              }
              event Panel Close? {
                n124 = event-data() -> ()  [unwired: 1 in, 4 out]
                n125 = Two Button Dialog(message="Exit Software?") -> (T button?=w379:bool)  [unwired: 2 in]
                n126 = case shown="True" w379 {
                  tunnel: [Main-state."Idle" Main-state."Exit"] -> w384
                  tunnel: w381 -> [w385 w389]
                  tunnel: [w385 w388] -> w380
                  frame False {
                  }
                  frame True {
                    n127 = control-ref of="This VI"() -> (w387:refnum<vi>)
                    n128 = call <vilib>:"Set Busy.vi"("error in (no error)"=w389, "VI reference (current VI)"=w387) -> ("error out"=w388:errorcluster)  [unwired: 8 in, 1 out]
                  }
                }
                n129 = event-data("Discard?"=TRUE) -> ()  [unwired: 1 in, 1 out]
              }
              event "Previous": Value Change {
                n130 = event-data() -> ()  [unwired: 1 in, 1 out]
                n131 = property on="Tab Array" class="Arr"(error in=w391) -> (error out=w394:errorcluster, "Index Values"=w401:u32[], "Number of Columns"=w398:u32)  [unwired: 1 in, 1 out]
                n132 = Subtract(x=w398, y=u32 12) -> (x-y=w396:u32)
                n133 = Increment(x=w401) -> (x+1=w395:u32[])
                n134 = Index Array(array=w395) -> (element=w400:u32)  [unwired: 1 in]
                n135 = property on="Tab Array" class="Arr"(error in=w394, "Index Values"=w395) -> (error out=w393:errorcluster)  [unwired: 1 in, 1 out]
                n136 = Equal?(x=w396, y=w400) -> (x = y?=w399:bool)
                n137 = case shown="True" w399 {
                  tunnel: w393 -> [w405 w409]
                  tunnel: [w404 w407] -> w392
                  frame False {
                    n138 = property on="Next" class="Bool"(error in=w405, "Visible"=TRUE) -> (error out=w404:errorcluster)  [unwired: 1 in, 1 out]
                  }
                  frame True {
                    n139 = property on="Next" class="Bool"(error in=w409, "Visible"=TRUE) -> (error out=w408:errorcluster)  [unwired: 1 in, 1 out]
                    n140 = property on="Previous" class="Bool"(error in=w408, "Visible"=FALSE) -> (error out=w407:errorcluster)  [unwired: 1 in, 1 out]
                  }
                }
              }
              event "Next": Value Change {
                n141 = event-data() -> ()  [unwired: 1 in, 1 out]
                n142 = property on="Tab Array" class="Arr"(error in=w412) -> (error out=w415:errorcluster, "Index Values"=w422:u32[], "Number of Columns"=w419:u32)  [unwired: 1 in, 1 out]
                n143 = Subtract(x=w419, y=u32 12) -> (x-y=w417:u32)
                n144 = Increment(x=w422) -> (x+1=w416:u32[])
                n145 = Index Array(array=w416) -> (element=w421:u32)  [unwired: 1 in]
                n146 = property on="Tab Array" class="Arr"(error in=w415, "Index Values"=w416) -> (error out=w414:errorcluster)  [unwired: 1 in, 1 out]
                n147 = Equal?(x=w417, y=w421) -> (x = y?=w420:bool)
                n148 = case shown="True" w420 {
                  tunnel: w414 -> [w426 w431]
                  tunnel: [w425 w428] -> w413
                  frame False {
                    n149 = property on="Previous" class="Bool"(error in=w426, "Visible"=TRUE) -> (error out=w425:errorcluster)  [unwired: 1 in, 1 out]
                  }
                  frame True {
                    n150 = property on="Previous" class="Bool"(error in=w431, "Visible"=TRUE) -> (error out=w429:errorcluster)  [unwired: 1 in, 1 out]
                    n151 = property on="Next" class="Bool"(error in=w429, "Visible"=FALSE) -> (error out=w428:errorcluster)  [unwired: 1 in, 1 out]
                  }
                }
              }
              event Value Change {
                n152 = event-data() -> ("NewVal"=w443:T5)  [unwired: 1 in]
                n153 = call "Main - Parse Data Tab (SubVI).vi"("NewVal"=w443) -> ("Bg"=w434:bool[], "Ok"=w447:bool[], "Cancel"=w444:bool[], "Tab"=w449:T16, "Run Test"=w433:refnum<vi>[])  [unwired: 6 in]
                n154 = Search 1D Array(1D array=w444, element=TRUE) -> (index of element=w448:i32)  [unwired: 1 in]
                n155 = Search 1D Array(1D array=w447, element=TRUE) -> (index of element=w450:i32)  [unwired: 1 in]
                n156 = Search 1D Array(1D array=w434, element=TRUE) -> (index of element=w452:i32)  [unwired: 1 in]
                n157 = case shown="0, Default" w450 {
                  selector: w450 -> [w457 _]
                  tunnel: w448 -> [_ w474]
                  tunnel: w449 -> [w462 w473]
                  tunnel: [w461 w472] -> w442
                  tunnel: w452 -> [_ w471]
                  tunnel: w441 -> [w459 w470]
                  tunnel: [w460 w469] -> w440
                  tunnel: w433 -> [w458 _]
                  tunnel: [w455 w468] -> w436
                  tunnel: [Main-state."Event" w467] -> w435
                  frame 0, Default {
                    # "Open Sub Panel"
                    n158 = in-place {
                      in-place-border: [w463] -> w455
                      n159 = in-place-array #1(w462, w457) -> (w466:T1)
                      n160 = Bundle By Name(cluster=w466, "Bg"=TRUE) -> (w464:T1)
                      n161 = Unbundle By Name(w464) -> ("fileid"=w463:string)
                      n162 = in-place-array #1(w464) -> (w461:T16)  [unwired: 1 out]
                    }
                    n163 = Index Array(array=w458, index=w457) -> (element=w456:refnum<vi>)
                    n164 = invoke on="Main Panel" class="SubPnl" method="Insert VI"(error in=w459, "VI Ref"=w456) -> (error out=w460:errorcluster)  [unwired: 2 in, 3 out]
                    n165 = local write "Close Panel"(T1 {"String"="", "Cancel Button"=FALSE, "OK Button"=FALSE, "Bg"=FALSE, "RunTest"=refnum, "fileid"="", "Stop"=FALSE, "Run"=FALSE, "Status"=""} ("Close Panel")) -> ()
                  }
                  frame -1 {
                    n166 = case shown="0, Default" w474 {
                      selector: w474 -> [w492 _]
                      tunnel: w473 -> [w494 w508]
                      tunnel: [w493 w508] -> w472
                      tunnel: w471 -> [w489 _]
                      tunnel: w470 -> [w485 w507]
                      tunnel: [w483 w507] -> w469
                      tunnel: [w477 "" ("fileid")] -> w468
                      tunnel: [Main-state."Event" Main-state."Idle"] -> w467
                      frame 0, Default {
                        n167 = Delete From Array(array=w494, index=w492) -> (deleted portion=→"Close Panel":T1, array with subset deleted=w491:T16)  [unwired: 1 in]
                        n168 = Decrement(x=w489) -> (x-1=w488:i32)
                        n169 = Decrement(x=w492) -> (x-1=w490:i32)
                        n170 = Equal?(x=w492, y=w489) -> (x = y?=w480:bool)
                        n171 = Select(t=w490, s=w480, f=w488) -> (s? t:f=w482:i32)
                        n172 = Empty Array?(array=w491) -> (empty?=w479:bool)
                        n173 = in-place {
                          in-place-border: [w501] -> w481
                          in-place-border: [w500] -> w477
                          n174 = in-place-array #2(w491, w482) -> (w504:T1)
                          n175 = Bundle By Name(cluster=w504, "Bg"=TRUE) -> (w502:T1)
                          n176 = Unbundle By Name(w502) -> ("fileid"=w500:string, "RunTest"=w501:refnum<vi>)
                          n177 = in-place-array #2(w502) -> (w493:T16)  [unwired: 1 out]
                        }
                        n178 = Array Size(array=w491) -> (size(s)=w487:i32)
                        n179 = Not(x=w479) -> (.not. x?=w486:bool)
                        n180 = property on="Tab Array" class="Arr"(error in=w485, "Number of Columns"=w487, "Visible"=w486) -> (error out=w484:errorcluster)  [unwired: 1 in, 1 out]
                        n181 = Or(x=w479, y=w480) -> (x .or. y?=w478:bool)
                        n182 = case shown="True" w478 {
                          tunnel: w484 -> [w495 w499]
                          tunnel: [w495 w497] -> w483
                          tunnel: w481 -> [_ w496]
                          frame False {
                          }
                          frame True {
                            n183 = invoke on="Main Panel" class="SubPnl" method="Remove VI"(error in=w499) -> (error out=w498:errorcluster)  [unwired: 2 in, 2 out]
                            n184 = invoke on="Main Panel" class="SubPnl" method="Insert VI"(error in=w498, "VI Ref"=w496) -> (error out=w497:errorcluster)  [unwired: 2 in, 3 out]
                          }
                        }
                      }
                      frame -1 {
                      }
                    }
                  }
                }
                n185 = Bundle By Name(cluster=w437, "FileId"=w436) -> (w438:T10)
                n186 = local write "Tab Array"(w442) -> ()
                n187 = call <vilib>:"Clear Errors.vi"("error in (no error)"=w440) -> ("error out"=w439:errorcluster)  [unwired: 5 in, 1 out]
              }
              event User Event {
                n188 = event-data() -> ("RunTest"=w514:refnum<vi>, "Name"=w511:string, "FileId"=w510:string, "Status"=w509:string)  [unwired: 1 in]
                n189 = Empty Array?(array="Tab Array") -> (empty?=w518:bool)
                n190 = for {
                  tunnel: "Tab Array" -> [w560] mode=indexing
                  tunnel: [w562] -> w520 mode=indexing
                  tunnel: [w559] -> w513 mode=indexing
                  n191 = Unbundle By Name(w560) -> ("RunTest"=w559:refnum<vi>)
                  n192 = Bundle By Name(cluster=w560, "Cancel Button"=FALSE, "OK Button"=FALSE, "Bg"=FALSE) -> (w562:T1)
                }
                n193 = case shown="True" w518 {
                  tunnel: [w566 0] -> w519
                  tunnel: "Tab Array" -> [w567 _]
                  tunnel: [w565 w569] -> w521
                  tunnel: w515 -> [w565 w568]
                  frame False {
                    n194 = Array Size(array=w567) -> (size(s)=w566:i32)
                  }
                  frame True {
                    n195 = property on="Tab Array" class="Arr"(error in=w568, "Visible"=TRUE) -> (error out=w569:errorcluster)  [unwired: 1 in, 1 out]
                  }
                }
                n196 = Search 1D Array(1D array=w513, element=w514) -> (index of element=w512:i32)  [unwired: 1 in]
                n197 = case shown="-1" w512 {
                  selector: w512 -> [w529 _]
                  tunnel: w521 -> [w527 w554]
                  tunnel: w520 -> [w530 w550]
                  tunnel: w519 -> [_ w545]
                  tunnel: [w526 w546] -> w516
                  tunnel: w514 -> [_ w542]
                  tunnel: w511 -> [w525 w544]
                  tunnel: w510 -> [_ w541]
                  tunnel: w509 -> [w524 w538]
                  frame 0, Default {
                    n198 = in-place {
                      in-place-border: w525 -> [w533]
                      in-place-border: w524 -> [w531]
                      n199 = in-place-array #3(w530, w529) -> (w536:T1)
                      n200 = Bundle By Name(cluster=w536, "OK Button"=TRUE, "Bg"=TRUE, "String"=w533, "Status"=w531) -> (w534:T1)
                      n201 = in-place-array #3(w534) -> (w528:T16)  [unwired: 1 out]
                    }
                    n202 = property on="Tab Array" class="Arr"(error in=w527, "Val(Sgnl)"=w528) -> (error out=w526:errorcluster)  [unwired: 1 in, 1 out]
                  }
                  frame -1 {
                    w547 = 12 ("y")
                    n203 = Increment(x=w545) -> (x+1=w552:i32)
                    n204 = Greater?(x=w552, y=w547) -> (0:w548:bool)
                    n205 = Subtract(x=w552, y=w547) -> (x-y=w549:i32)
                    n206 = Bundle By Name(cluster=T1 {"String"="", "Cancel Button"=FALSE, "OK Button"=FALSE, "Bg"=FALSE, "RunTest"=refnum, "fileid"="", "Stop"=FALSE, "Run"=FALSE, "Status"=""} ("Cluster"), "OK Button"=TRUE, "RunTest"=w542, "String"=w544, "fileid"=w541, "Status"=w538) -> (w543:T1)
                    n207 = Build Array(w549) -> (w551:i32[])
                    n208 = property on="Tab Array" class="Arr"(error in=w554, "Number of Columns"=w552, "Index Values"=w551) -> (error out=w553:errorcluster)  [unwired: 1 in, 1 out]
                    n209 = Insert Into Array(array=w550, index=w545, new element=w543) -> (w540:T16)
                    n210 = case shown="False" w548 {
                      tunnel: w553 -> [w555 w557]
                      tunnel: [w555 w556] -> w546
                      frame False {
                      }
                      frame True {
                        n211 = property on="Previous" class="Bool"(error in=w557, "Visible"=TRUE) -> (error out=w556:errorcluster)  [unwired: 1 in, 1 out]
                      }
                    }
                    n212 = property on="Tab Array" class="Arr"("Val(Sgnl)"=w540) -> ()  [unwired: 2 in, 2 out]
                  }
                }
              }
              event "EventSwitch": Value Change {
                n213 = event-data() -> ("NewVal"=w572:bool)  [unwired: 1 in]
                n214 = Select(t=i16 140, s=w572, f=i16 55 ("y")) -> (s? t:f=w580:i16)
                n215 = Subtract(x=w583, y=w580) -> (x-y=w578:i16)
                n216 = property on="Splitter 10" class="Splitter"(error in=w579, "Position"=w578) -> (error out=w574:errorcluster)  [unwired: 1 in, 1 out]
                n217 = Select(t="Event v" ("Caption.Text"), s=w572, f="Event ^" ("Caption.Text")) -> (s? t:f=w577:string)
                n218 = property on="Event" class="Str"(error in=w574, "Caption.Text"=w577) -> (error out=w573:errorcluster)  [unwired: 1 in, 1 out]
              }
            }
          }
          frame "Change page" {
            n219 = Unbundle By Name(w594) -> ("Module Ref"=w589:refnum<vi>[], "Side Name"=w586:string)
            n220 = call "Main - Search VI Ref (SubVI).vi"("Error In"=w592, "VI Name to Search"=w586, "VI Refs"=w589) -> ("Error Out"=w591:errorcluster, "VI Ref Found"=w587:refnum<vi>, "Found?"=w590:bool)  [unwired: 6 in]
            n221 = case shown="\"Modules - Explorer.vi\"" w586 {
              tunnel: [w600 w610] -> w596
              tunnel: w591 -> [w599 w609]
              tunnel: w590 -> [w598 w608]
              tunnel: w587 -> [w597 w607]
              frame Default {
                n222 = case shown="True" w598 {
                  tunnel: [w601 w604] -> w600
                  tunnel: w597 -> [_ w603]
                  tunnel: w599 -> [w601 w602]
                  frame False {
                  }
                  frame True {
                    n223 = invoke class="VI" method="FP.Open"(reference=w603, error in=w602, "Activate"=TRUE ("Activate?"), "State"=T6."Standard") -> (error out=w604:errorcluster)  [unwired: 1 in, 4 out]
                  }
                }
              }
              frame "Modules - Explorer.vi" {
                n224 = case shown="True" w608 {
                  tunnel: [w611 w618] -> w610
                  tunnel: w607 -> [_ w613]
                  tunnel: w609 -> [w611 w617]
                  frame False {
                  }
                  frame True {
                    n225 = invoke on="Sub Panel" class="SubPnl" method="Remove VI"(error in=w617) -> (error out=w615:errorcluster)  [unwired: 2 in, 2 out]
                    n226 = property class="VI"(reference=w613, error in=w615, "Front Panel.WinBounds"=T13 {"Left"=1146, "Top"=168, "Right"=1492, "Bottom"=898} ("Front Panel Window:Window Bounds")) -> (reference out=w614:refnum<vi>, error out=w612:errorcluster)
                    n227 = invoke class="VI" method="FP.Open"(reference=w614, error in=w612, "Activate"=TRUE ("Activate?"), "State"=T6."Standard") -> (error out=w618:errorcluster)  [unwired: 1 in, 4 out]
                  }
                }
              }
            }
            n228 = call <vilib>:"Clear Errors.vi"("error in (no error)"=w596) -> ("error out"=w595:errorcluster)  [unwired: 5 in, 1 out]
          }
          frame "Manual Control" {
            (unwired) "Modules - Manual Control.vit"
            w631 = "Main" ("element")
            n229 = call "Main - Manual Control Deamon Ref (FGV).vi"("Action"=FGV_States."Read", "error in"=w630) -> ("error out"=w623:errorcluster, "Name out"=w632:string[], "Ref out"=w633:refnum<vi>[])  [unwired: 7 in]
            n230 = Build Path(base path=w626, name or relative path="Modules") -> (appended path=w629:path)
            n231 = call "Main - Page eFGV.vi"("eFGV States"=eFGV_States."Write", "error in (no error)"=w623, "Page In"=T12."Machine Control") -> ("error out"=w622:errorcluster)  [unwired: 6 in, 2 out]
            n232 = Search 1D Array(1D array=w632, element=w631) -> (index of element=w634:i32)  [unwired: 1 in]
            n233 = Build Path(base path=w629, name or relative path="Modules - Manual Control V2.vit") -> (appended path=w627:path)
            n234 = case shown="-1" w634 {
              selector: w634 -> [w645 _]
              tunnel: w622 -> [w644 w668]
              tunnel: [w643 w663] -> w635
              tunnel: w633 -> [w646 w659]
              tunnel: w632 -> [_ w662]
              tunnel: w631 -> [_ w661]
              tunnel: w627 -> [_ w651]
              frame 0, Default {
                n235 = Index Array(array=w646, index=w645) -> (element=w642:refnum<vi>)
                n236 = invoke class="VI" method="FP.Open"(reference=w642, error in=w644, "Activate"=TRUE ("Activate?"), "State"=T6."Standard") -> (error out=w643:errorcluster)  [unwired: 1 in, 4 out]
              }
              frame -1 {
                n237 = Open VI Reference(vi path=w651, error in (no error)=w668) -> (vi reference=w667:refnum<vi>, error out=w666:errorcluster)  [unwired: 4 in]
                n238 = Build Array (concatenate)(w662, w661) -> (w658:string[])
                n239 = invoke class="VI" method="Ctrl Val.Set"(reference=w667, error in=w666, "Control Name"="Device Name", "Value"="" ("Control Name")) -> (reference out=w650:refnum<vi>, error out=w648:errorcluster)  [unwired: 1 in, 3 out]
                n240 = invoke class="VI" method="Run VI"(reference=w650, error in=w648, "Wait until done"=FALSE ("Wait Until Done"), "Auto Dispose Ref"=FALSE ("Auto Dispose Reference")) -> (reference out=w649:refnum<vi>, error out=w647:errorcluster)  [unwired: 1 in, 3 out]
                n241 = invoke class="VI" method="FP.Open"(reference=w649, error in=w647, "Activate"=TRUE ("Activate?"), "State"=T6."Standard") -> (error out=w655:errorcluster)  [unwired: 1 in, 4 out]
                n242 = Build Array (concatenate)(w659, w649) -> (w660:refnum<vi>[])
                n243 = call "Main - Manual Control Deamon Ref (FGV).vi"("Action"=FGV_States."Write", "error in"=w655, "Name"=w658, "Ref in"=w660) -> ("error out"=w663:errorcluster)  [unwired: 5 in, 2 out]
              }
            }
          }
          frame "NewTest" {
            n244 = Greater?(x=w671, y=i16 1900) -> ()  [unwired: 1 out]
            n245 = Build Path(base path=w682, name or relative path="Modules") -> (appended path=w685:path)
            n246 = Build Path(base path=w685, name or relative path="Modules - Run Test with Config.vit") -> (appended path=w683:path)
            n247 = Open VI Reference(vi path=w683, error in (no error)=w675) -> (vi reference=w673:refnum<vi>, error out=w672:errorcluster)  [unwired: 4 in]
            n248 = invoke class="VI" method="Run VI"(reference=w673, error in=w672, "Wait until done"=FALSE ("Wait Until Done"), "Auto Dispose Ref"=FALSE ("Auto Dispose Reference")) -> (reference out=w677:refnum<vi>, error out=w676:errorcluster)  [unwired: 1 in, 3 out]
            n249 = invoke class="VI" method="FP.Open"(reference=w677, error in=w676, "Activate"=TRUE ("Activate?"), "State"=T6."Standard") -> (error out=w674:errorcluster)  [unwired: 1 in, 4 out]
          }
          frame "sidepanel" {
            n250 = Unbundle By Name(w697) -> ("Module Ref"=w694:refnum<vi>[], "pin"=w690:bool)
            n251 = call "Main - Search VI Ref (SubVI).vi"("Error In"=w695, "VI Name to Search"="Modules - Explorer.vi", "VI Refs"=w694) -> ("Error Out"=w696:errorcluster, "VI Ref Found"=w692:refnum<vi>, "Found?"=w691:bool)  [unwired: 6 in]
            n252 = case shown="False" w690 {
              tunnel: [w705 w718] -> w698
              tunnel: w696 -> [w704 w717]
              tunnel: w692 -> [w703 w715]
              tunnel: w691 -> [w702 w716]
              tunnel: w689 -> [w701 w714]
              frame True {
                n253 = case shown="True" w702 {
                  tunnel: [w706 w713] -> w705
                  tunnel: w704 -> [w706 w710]
                  tunnel: w703 -> [_ w712]
                  tunnel: w701 -> [_ w709]
                  frame False {
                  }
                  frame True {
                    n254 = Subtract(x=w709, y=i16 350) -> (x-y=w707:i16)
                    n255 = property on="Splitter 9" class="Splitter"(error in=w710, "Position"=w707) -> (error out=w711:errorcluster)  [unwired: 1 in, 1 out]
                    n256 = invoke on="Sub Panel" class="SubPnl" method="Insert VI"(error in=w711, "VI Ref"=w712) -> (error out=w713:errorcluster)  [unwired: 2 in, 3 out]
                  }
                }
              }
              frame False {
                n257 = case shown="True" w716 {
                  tunnel: [w719 w731] -> w718
                  tunnel: w717 -> [w719 w732]
                  tunnel: w715 -> [_ w726]
                  tunnel: w714 -> [_ w722]
                  frame False {
                  }
                  frame True {
                    n258 = invoke on="Sub Panel" class="SubPnl" method="Remove VI"(error in=w732) -> (error out=w724:errorcluster)  [unwired: 2 in, 2 out]
                    n259 = Subtract(x=w722, y=i16 42) -> (x-y=w720:i16)
                    n260 = property on="Splitter 9" class="Splitter"(error in=w724, "Position"=w720) -> (error out=w723:errorcluster)  [unwired: 1 in, 1 out]
                    n261 = property class="VI"(reference=w726, error in=w723, "Front Panel.WinBounds"=T13 {"Left"=1146, "Top"=168, "Right"=1492, "Bottom"=898} ("Front Panel Window:Window Bounds")) -> (reference out=w727:refnum<vi>, error out=w725:errorcluster)
                    n262 = invoke class="VI" method="FP.Open"(reference=w727, error in=w725, "Activate"=TRUE ("Activate?"), "State"=T6."Standard") -> (error out=w731:errorcluster)  [unwired: 1 in, 4 out]
                  }
                }
              }
            }
          }
          frame "Event" {
            n263 = Unbundle By Name(w740) -> ("FileId"=w739:string)
            n264 = local read "Close Panel"() -> (w738:T1)
            n265 = call "Main - Event Log (eFGV).vi"("Action"=eFGV_States."Read", "error in"=w741, "Fileid"=w739) -> ("error out"=w735:errorcluster, "Data Out"=→"Event":string)  [unwired: 5 in, 2 out]
            n266 = Unbundle By Name(w738) -> ("fileid"=w733:string, "RunTest"=w734:refnum<vi>)
            n267 = Empty String/Path?(string/path=w733) -> (empty?=w737:bool)
            n268 = case shown="False" w737 {
              tunnel: [w752 w797] -> w736
              tunnel: w735 -> [w763 w797]
              tunnel: w734 -> [w746 _]
              tunnel: w733 -> [w755 _]
              frame False {
                n269 = property class="VI"(reference=w746, error in=w763) -> (error out=w762:errorcluster, "Front Panel.Title"=w749:string)  [unwired: 1 out]
                n270 = Search and Replace String(input string=w749, search string="Complete") -> (number of replacements=w748:i32)  [unwired: 6 in, 3 out]
                n271 = Search and Replace String(input string=w749, search string="Idle", error in=w762) -> (number of replacements=w760:i32, error out=w754:errorcluster)  [unwired: 5 in, 2 out]
                n272 = Bundle By Name(cluster=cluster{"action":string, "id":string} {"action"="delete", "id"=""}, "id"=w755) -> (w753:cluster{"action":string, "id":string})
                n273 = Greater Than 0?(x=w748) -> (x > 0?=w747:bool)
                n274 = Greater Than 0?(x=w760) -> (x > 0?=w751:bool)
                n275 = case shown="False" w751 {
                  tunnel: "http://localhost/filename.php" ("url") -> [_ w796]
                  tunnel: "Content-Type" ("header") -> [_ w793]
                  tunnel: "application/json" ("value") -> [_ w792]
                  tunnel: w754 -> [w766 w789]
                  tunnel: w753 -> [_ w787]
                  tunnel: [w765 w781] -> w752
                  tunnel: w747 -> [w767 _]
                  tunnel: w746 -> [w764 _]
                  frame False {
                    n276 = case shown="True" w767 {
                      tunnel: w766 -> [w768 w777]
                      tunnel: [w768 w770] -> w765
                      tunnel: w764 -> [_ w769]
                      frame False {
                      }
                      frame True {
                        n277 = call "Runtest - Deamon Ref (FGV).vi"("Action"=FGV_States."Read", "error in"=w777) -> ("error out"=w778:errorcluster, "Name out"=w775:string[], "Ref out"=w776:refnum<vi>[])  [unwired: 7 in]
                        n278 = Search 1D Array(1D array=w776, element=w769) -> (index of element=w774:i32)  [unwired: 1 in]
                        n279 = Delete From Array(array=w776, index=w774) -> (array with subset deleted=w772:refnum<vi>[])  [unwired: 1 in, 1 out]
                        n280 = Delete From Array(array=w775, index=w774) -> (array with subset deleted=w773:string[])  [unwired: 1 in, 1 out]
                        n281 = call "Runtest - Deamon Ref (FGV).vi"("Action"=FGV_States."Write", "error in"=w778, "Name"=w773, "Ref in"=w772) -> ("error out"=w771:errorcluster)  [unwired: 5 in, 2 out]
                        n282 = invoke class="VI" method="Abort VI"(reference=w769, error in=w771) -> (error out=w770:errorcluster)  [unwired: 1 in, 2 out]
                      }
                    }
                  }
                  frame True {
                    n283 = Flatten To JSON(anything=w787, error in (no error)=w789) -> (JSON string=w786:string, 11:w788:errorcluster)  [unwired: 1 in]
                    n284 = call <vilib>:"OpenHandle.vi"("error in (no error)"=w788) -> ("client handle out"=w794:T17, "error out"=w795:errorcluster)  [unwired: 13 in]
                    n285 = call <vilib>:"AddHeader.vi"("client handle"=w794, "header"=w793, "value"=w792, "error in (no error)"=w795) -> ("client handle out"=w790:T17, "error out"=w791:errorcluster)  [unwired: 10 in]
                    n286 = call-poly <vilib>:"POST.vi"("client handle"=w790, "url"=w796, "buffer"=w786, "error in (no error)"=w791) -> ("client handle out"=w784:T17, "error out"=w785:errorcluster)  [unwired: 8 in, 2 out]
                    n287 = call <vilib>:"CloseHandle.vi"("client handle"=w784, "error in (no error)"=w785) -> ("error out"=w782:errorcluster)  [unwired: 13 in]
                    n288 = call "Main - Update Tree (eFGV).vi"("Action"=eFGV_States."Write", "error in"=w782) -> ("error out"=w781:errorcluster)  [unwired: 7 in, 2 out]
                  }
                }
              }
              frame True {
              }
            }
          }
          frame "Emergency" {
            n289 = local read "Tab Array"() -> (w803:T5)
            n290 = for {
              tunnel: w803 -> [w822] mode=indexing
              shift-right: [w820] -> w802
              shift-left: w799 -> [w819]
              n291 = Unbundle By Name(w822) -> ("fileid"=w816:string)
              n292 = Concatenate Strings("Emergency", " - " ("string"), w816) -> (w815:string)
              n293 = call "Main - EndStage (eFGV).vi"("Action"=eFGV_States."Write", "error in"=w819, "Endstage In"=w815) -> ("error out"=w820:errorcluster)  [unwired: 6 in, 2 out]
            }
            n294 = global read "Global - IP Address.vi" "IP"() -> (w801:string[])
            n295 = for {
              shift-right: [w808] -> w800
              shift-left: w802 -> [w809]
              tunnel: w801 -> [w807] mode=indexing
              n296 = case shown="\"True\", Default" w807 {
                selector: w807 -> [_ w811]
                tunnel: w809 -> [w810 w813]
                tunnel: [w810 w812] -> w808
                frame "" {
                }
                frame "True", Default {
                  n297 = call "Communication - Send Command Read.vi"("error in (no error)"=w813, "Action"=UDP_-_Command."Stop", "Device IP Address"=w811) -> ("error out"=w812:errorcluster)  [unwired: 8 in]
                }
              }
            }
            n298 = call <vilib>:"Clear Errors.vi"("error in (no error)"=w800) -> ("error out"=w798:errorcluster)  [unwired: 5 in, 1 out]
          }
          frame "Exit" {
            n299 = Unbundle By Name(w856) -> ("Module Ref"=w853:refnum<vi>[])
            n300 = global read "Global - IP Address.vi" "IP"() -> (w844:string[])
            n301 = global read "Global - Handle V1.vi" "Handle"() -> (w825:refnum<visa-resource-name>[])
            n302 = for {
              shift-right: [w861] -> w823
              shift-left: w824 -> [w864]
              tunnel: w825 -> [w862] mode=indexing
              n303 = VISA Close(VISA resource name=w862, error in (no error)=w864) -> (error out=w863:errorcluster)
              n304 = call <vilib>:"Clear Errors.vi"("error in (no error)"=w863) -> ("error out"=w861:errorcluster)  [unwired: 5 in, 1 out]
            }
            n305 = for {
              tunnel: w844 -> [w879] mode=indexing
              shift-right: [w881] -> w843
              shift-left: w823 -> [w880]
              n306 = call "Communication - Send Command Read.vi"("Bypass?"=FALSE, "error in (no error)"=w880, "Action"=UDP_-_Command."Stop", "Device IP Address"=w879) -> ("error out"=w881:errorcluster)  [unwired: 7 in]
            }
            n307 = global read "Global - Handle.vi" "Handle"() -> (w842:T18)
            n308 = for {
              shift-right: [w872] -> w832
              shift-left: w843 -> [w876]
              tunnel: w842 -> [w874] mode=indexing
              n309 = Unbundle By Name(w874) -> ("UDP ref"=w873:refnum<k16>)
              n310 = UDP Close(connection ID=w873, 8:w876) -> (error out=w875:errorcluster)  [unwired: 1 out]
              n311 = call <vilib>:"Clear Errors.vi"("error in (no error)"=w875) -> ("error out"=w872:errorcluster)  [unwired: 5 in, 1 out]
            }
            n312 = call <vilib>:"Application Directory.vi"() -> ("Application Directory"=w836:path)
            n313 = global read "Global - Data UDP.vi" "V1"() -> (w830:bool)
            n314 = Build Path(base path=w836, name or relative path="Data\\stop_ping.txt") -> (appended path=w834:path)
            n315 = case shown="False" w830 {
              tunnel: w834 -> [w870 _]
              tunnel: T15."create" ("operation (0:open)") -> [w869 _]
              tunnel: w832 -> [w866 w871]
              tunnel: [w865 w871] -> w831
              frame False {
                n316 = Open/Create/Replace File(file path (use dialog)=w870, error in=w866, operation (0:open)=w869) -> (refnum out=w868:refnum<file>, error out=w867:errorcluster)  [unwired: 3 in, 1 out]
                n317 = Close File(refnum=w868, error in=w867) -> (error out=w865:errorcluster)  [unwired: 1 out]
              }
              frame True {
              }
            }
            n318 = call "Main - Manual Control Deamon Ref (FGV).vi"("Action"=FGV_States."Read", "error in"=w831) -> ("error out"=w840:errorcluster, "Ref out"=w839:refnum<vi>[])  [unwired: 7 in, 1 out]
            n319 = call <vilib>:"Application Directory.vi"() -> ("Application Directory"=w829:path)
            n320 = Build Path(base path=w829, name or relative path="Data\\ping_results.csv") -> (appended path=w827:path)
            n321 = call "General - Exit eFGV.vi"("eFGV States"=eFGV_States."Write", "error in (no error)"=w840, "Exit In"=TRUE) -> ("error out"=w851:errorcluster)  [unwired: 6 in, 2 out]
            n322 = call "Runtest - Deamon Ref (FGV).vi"("Action"=FGV_States."Read", "error in"=w851) -> ("error out"=w854:errorcluster, "Ref out"=w838:refnum<vi>[])  [unwired: 7 in, 1 out]
            n323 = Build Array (concatenate)(w853, w839, w838) -> (w852:refnum<vi>[])
            n324 = for {
              tunnel: w852 -> [w882] mode=indexing
              shift-right: [w883] -> w845
              shift-left: w854 -> [w885]
              n325 = invoke class="VI" method="Abort VI"(reference=w882, error in=w885) -> (error out=w884:errorcluster)  [unwired: 1 in, 2 out]
              n326 = call <vilib>:"Clear Errors.vi"("error in (no error)"=w884) -> ("error out"=w883:errorcluster)  [unwired: 5 in, 1 out]
            }
            n327 = Delete(path (use dialog)=w827) -> (error out=→"error out":errorcluster)  [unwired: 4 in, 2 out]
            n328 = control-ref of="This VI"() -> (w850:refnum<vi>)
            n329 = invoke class="VI" method="FP.Close"(reference=w850, error in=w845) -> (reference out=w847:refnum<vi>, error out=w849:errorcluster)  [unwired: 1 in, 1 out]
            n330 = call <vilib>:"Unset Busy.vi"("error in (no error)"=w849, "VI reference (current VI)"=w847) -> ("error out"=w848:errorcluster)  [unwired: 9 in]
          }
        }
      }
      frame Error {
        n331 = call <vilib>:"Clear Errors.vi"("error in (no error)"=w891) -> ("error out"=w888:errorcluster)  [unwired: 5 in, 1 out]
        n332 = Wait (ms)(milliseconds to wait=u32 100) -> ()  [unwired: 1 out]
      }
    }
  }
  n333 = case shown="No Error" w24 {
    frame No Error {
      w902 = string[] [] ("SN")
      n334 = global write "Global - Done.vi" "Done"(bool[] [FALSE, FALSE, FALSE, FALSE, FALSE, FALSE, FALSE, FALSE, FALSE, FALSE, FALSE, FALSE, FALSE, FALSE, FALSE, FALSE] ("Done")) -> ()
      n335 = global write "Global - Channel.vi" "Data"(T21 [{"Channels"={"Ch1"=0.0, "Ch2"=0.0, "Ch3"=0.0, "Ch4"=0.0, "Ch5"=0.0, "Ch6"=0.0, "Ch7"=0.0, "Ch8"=0.0, "Ch9"=0.0, "Ch10"=0.0, "Ch11"=0.0, "Ch12"=0.0, "Ch13"=0.0, "Ch14"=0.0, "Ch15"=0.0, "Ch16"=0.0}, "Event"=0, "Status"=0, ""}, {"Channels"={"Ch1"=0.0, "Ch2"=0.0, "Ch3"=0.0, "Ch4"=0.0, "Ch5"=0.0, "Ch6"=0.0, "Ch7"=0.0, "Ch8"=0.0, "Ch9"=0.0, "Ch10"=0.0, "Ch11"=0.0, "Ch12"=0.0, "Ch13"=0.0, "Ch14"=0.0, "Ch15"=0.0, "Ch16"=0.0}, "Event"=0, "Status"=0, ""}, {"Channels"={"Ch1"=0.0, "Ch2"=0.0, "Ch3"=0.0, "Ch4"=0.0, "Ch5"=0.0, "Ch6"=0.0, "Ch7"=0.0, "Ch8"=0.0, "Ch9"=0.0, "Ch10"=0.0, "Ch11"=0.0, "Ch12"=0.0, "Ch13"=0.0, "Ch14"=0.0, "Ch15"=0.0, "Ch16"=0.0}, "Event"=0, "Status"=0, ""}, {"Channels"={"Ch1"=0.0, "Ch2"=0.0, "Ch3"=0.0, "Ch4"=0.0, "Ch5"=0.0, "Ch6"=0.0, "Ch7"=0.0, "Ch8"=0.0, "Ch9"=0.0, "Ch10"=0.0, "Ch11"=0.0, "Ch12"=0.0, "Ch13"=0.0, "Ch14"=0.0, "Ch15"=0.0, "Ch16"=0.0}, "Event"=0, "Status"=0, ""}, {"Channels"={"Ch1"=0.0, "Ch2"=0.0, "Ch3"=0.0, "Ch4"=0.0, "Ch5"=0.0, "Ch6"=0.0, "Ch7"=0.0, "Ch8"=0.0, "Ch9"=0.0, "Ch10"=0.0, "Ch11"=0.0, "Ch12"=0.0, "Ch13"=0.0, "Ch14"=0.0, "Ch15"=0.0, "Ch16"=0.0}, "Event"=0, "Status"=0, ""}, {"Channels"={"Ch1"=0.0, "Ch2"=0.0, "Ch3"=0.0, "Ch4"=0.0, "Ch5"=0.0, "Ch6"=0.0, "Ch7"=0.0, "Ch8"=0.0, "Ch9"=0.0, "Ch10"=0.0, "Ch11"=0.0, "Ch12"=0.0, "Ch13"=0.0, "Ch14"=0.0, "Ch15"=0.0, "Ch16"=0.0}, "Event"=0, "Status"=0, ""}, {"Channels"={"Ch1"=0.0, "Ch2"=0.0, "Ch3"=0.0, "Ch4"=0.0, "Ch5"=0.0, "Ch6"=0.0, "Ch7"=0.0, "Ch8"=0.0, "Ch9"=0.0, "Ch10"=0.0, "Ch11"=0.0, "Ch12"=0.0, "Ch13"=0.0, "Ch14"=0.0, "Ch15"=0.0, "Ch16"=0.0}, "Event"=0, "Status"=0, ""}, {"Channels"={"Ch1"=0.0, "Ch2"=0.0, "Ch3"=0.0, "Ch4"=0.0, "Ch5"=0.0, "Ch6"=0.0, "Ch7"=0.0, "Ch8"=0.0, "Ch9"=0.0, "Ch10"=0.0, "Ch11"=0.0, "Ch12"=0.0, "Ch13"=0.0, "Ch14"=0.0, "Ch15"=0.0, "Ch16"=0.0}, "Event"=0, "Status"=0, ""}, {"Channels"={"Ch1"=0.0, "Ch2"=0.0, "Ch3"=0.0, "Ch4"=0.0, "Ch5"=0.0, "Ch6"=0.0, "Ch7"=0.0, "Ch8"=0.0, "Ch9"=0.0, "Ch10"=0.0, "Ch11"=0.0, "Ch12"=0.0, "Ch13"=0.0, "Ch14"=0.0, "Ch15"=0.0, "Ch16"=0.0}, "Event"=0, "Status"=0, ""}, {"Channels"={"Ch1"=0.0, "Ch2"=0.0, "Ch3"=0.0, "Ch4"=0.0, "Ch5"=0.0, "Ch6"=0.0, "Ch7"=0.0, "Ch8"=0.0, "Ch9"=0.0, "Ch10"=0.0, "Ch11"=0.0, "Ch12"=0.0, "Ch13"=0.0, "Ch14"=0.0, "Ch15"=0.0, "Ch16"=0.0}, "Event"=0, "Status"=0, ""}, {"Channels"={"Ch1"=0.0, "Ch2"=0.0, "Ch3"=0.0, "Ch4"=0.0, "Ch5"=0.0, "Ch6"=0.0, "Ch7"=0.0, "Ch8"=0.0, "Ch9"=0.0, "Ch10"=0.0, "Ch11"=0.0, "Ch12"=0.0, "Ch13"=0.0, "Ch14"=0.0, "Ch15"=0.0, "Ch16"=0.0}, "Event"=0, "Status"=0, ""}, {"Channels"={"Ch1"=0.0, "Ch2"=0.0, "Ch3"=0.0, "Ch4"=0.0, "Ch5"=0.0, "Ch6"=0.0, "Ch7"=0.0, "Ch8"=0.0, "Ch9"=0.0, "Ch10"=0.0, "Ch11"=0.0, "Ch12"=0.0, "Ch13"=0.0, "Ch14"=0.0, "Ch15"=0.0, "Ch16"=0.0}, "Event"=0, "Status"=0, ""}, {"Channels"={"Ch1"=0.0, "Ch2"=0.0, "Ch3"=0.0, "Ch4"=0.0, "Ch5"=0.0, "Ch6"=0.0, "Ch7"=0.0, "Ch8"=0.0, "Ch9"=0.0, "Ch10"=0.0, "Ch11"=0.0, "Ch12"=0.0, "Ch13"=0.0, "Ch14"=0.0, "Ch15"=0.0, "Ch16"=0.0}, "Event"=0, "Status"=0, ""}, {"Channels"={"Ch1"=0.0, "Ch2"=0.0, "Ch3"=0.0, "Ch4"=0.0, "Ch5"=0.0, "Ch6"=0.0, "Ch7"=0.0, "Ch8"=0.0, "Ch9"=0.0, "Ch10"=0.0, "Ch11"=0.0, "Ch12"=0.0, "Ch13"=0.0, "Ch14"=0.0, "Ch15"=0.0, "Ch16"=0.0}, "Event"=0, "Status"=0, ""}, {"Channels"={"Ch1"=0.0, "Ch2"=0.0, "Ch3"=0.0, "Ch4"=0.0, "Ch5"=0.0, "Ch6"=0.0, "Ch7"=0.0, "Ch8"=0.0, "Ch9"=0.0, "Ch10"=0.0, "Ch11"=0.0, "Ch12"=0.0, "Ch13"=0.0, "Ch14"=0.0, "Ch15"=0.0, "Ch16"=0.0}, "Event"=0, "Status"=0, ""}, {"Channels"={"Ch1"=0.0, "Ch2"=0.0, "Ch3"=0.0, "Ch4"=0.0, "Ch5"=0.0, "Ch6"=0.0, "Ch7"=0.0, "Ch8"=0.0, "Ch9"=0.0, "Ch10"=0.0, "Ch11"=0.0, "Ch12"=0.0, "Ch13"=0.0, "Ch14"=0.0, "Ch15"=0.0, "Ch16"=0.0}, "Event"=0, "Status"=0, ""}] ("Data")) -> ()
      n336 = global write "Global - Data UDP.vi" "Channels"(T22 {"Ch1"=0.0, "Ch2"=0.0, "Ch3"=0.0, "Ch4"=0.0, "Ch5"=0.0, "Ch6"=0.0, "Ch7"=0.0, "Ch8"=0.0, "Ch9"=0.0, "Ch10"=0.0, "Ch11"=0.0, "Ch12"=0.0, "Ch13"=0.0, "Ch14"=0.0, "Ch15"=0.0, "Ch16"=0.0} ("Channels")) -> ()
      n337 = global write "Global - PID.vi" "PID"(T25 [{"SP"=0.0, "PV"=0.0, "kP"=0.0, "kI"=0.0, "kD"=0.0, "FF"=0.0, "Err Band"=0.0, "Max"=0, "Min"=0, "Ts"=0, "Out"=0, "Mode"=0}, {"SP"=0.0, "PV"=0.0, "kP"=0.0, "kI"=0.0, "kD"=0.0, "FF"=0.0, "Err Band"=0.0, "Max"=0, "Min"=0, "Ts"=0, "Out"=0, "Mode"=0}, {"SP"=0.0, "PV"=0.0, "kP"=0.0, "kI"=0.0, "kD"=0.0, "FF"=0.0, "Err Band"=0.0, "Max"=0, "Min"=0, "Ts"=0, "Out"=0, "Mode"=0}, {"SP"=0.0, "PV"=0.0, "kP"=0.0, "kI"=0.0, "kD"=0.0, "FF"=0.0, "Err Band"=0.0, "Max"=0, "Min"=0, "Ts"=0, "Out"=0, "Mode"=0}, {"SP"=0.0, "PV"=0.0, "kP"=0.0, "kI"=0.0, "kD"=0.0, "FF"=0.0, "Err Band"=0.0, "Max"=0, "Min"=0, "Ts"=0, "Out"=0, "Mode"=0}, {"SP"=0.0, "PV"=0.0, "kP"=0.0, "kI"=0.0, "kD"=0.0, "FF"=0.0, "Err Band"=0.0, "Max"=0, "Min"=0, "Ts"=0, "Out"=0, "Mode"=0}, {"SP"=0.0, "PV"=0.0, "kP"=0.0, "kI"=0.0, "kD"=0.0, "FF"=0.0, "Err Band"=0.0, "Max"=0, "Min"=0, "Ts"=0, "Out"=0, "Mode"=0}, {"SP"=0.0, "PV"=0.0, "kP"=0.0, "kI"=0.0, "kD"=0.0, "FF"=0.0, "Err Band"=0.0, "Max"=0, "Min"=0, "Ts"=0, "Out"=0, "Mode"=0}, {"SP"=0.0, "PV"=0.0, "kP"=0.0, "kI"=0.0, "kD"=0.0, "FF"=0.0, "Err Band"=0.0, "Max"=0, "Min"=0, "Ts"=0, "Out"=0, "Mode"=0}, {"SP"=0.0, "PV"=0.0, "kP"=0.0, "kI"=0.0, "kD"=0.0, "FF"=0.0, "Err Band"=0.0, "Max"=0, "Min"=0, "Ts"=0, "Out"=0, "Mode"=0}, {"SP"=0.0, "PV"=0.0, "kP"=0.0, "kI"=0.0, "kD"=0.0, "FF"=0.0, "Err Band"=0.0, "Max"=0, "Min"=0, "Ts"=0, "Out"=0, "Mode"=0}, {"SP"=0.0, "PV"=0.0, "kP"=0.0, "kI"=0.0, "kD"=0.0, "FF"=0.0, "Err Band"=0.0, "Max"=0, "Min"=0, "Ts"=0, "Out"=0, "Mode"=0}, {"SP"=0.0, "PV"=0.0, "kP"=0.0, "kI"=0.0, "kD"=0.0, "FF"=0.0, "Err Band"=0.0, "Max"=0, "Min"=0, "Ts"=0, "Out"=0, "Mode"=0}, {"SP"=0.0, "PV"=0.0, "kP"=0.0, "kI"=0.0, "kD"=0.0, "FF"=0.0, "Err Band"=0.0, "Max"=0, "Min"=0, "Ts"=0, "Out"=0, "Mode"=0}, {"SP"=0.0, "PV"=0.0, "kP"=0.0, "kI"=0.0, "kD"=0.0, "FF"=0.0, "Err Band"=0.0, "Max"=0, "Min"=0, "Ts"=0, "Out"=0, "Mode"=0}, {"SP"=0.0, "PV"=0.0, "kP"=0.0, "kI"=0.0, "kD"=0.0, "FF"=0.0, "Err Band"=0.0, "Max"=0, "Min"=0, "Ts"=0, "Out"=0, "Mode"=0}] ("PID")) -> ()
      n338 = global write "Global - Device.vi" "Device"(w902) -> ()
      n339 = global write "Global - Handle.vi" "Handle"(T18 [] ("Handle")) -> ()
      n340 = global write "Global - Test.vi" "Test"(T23 [{"Target Load"=0.0, "Target Disp"=0.0, "Rate"=0.0, "Speed"=0.0}, {"Target Load"=0.0, "Target Disp"=0.0, "Rate"=0.0, "Speed"=0.0}, {"Target Load"=0.0, "Target Disp"=0.0, "Rate"=0.0, "Speed"=0.0}, {"Target Load"=0.0, "Target Disp"=0.0, "Rate"=0.0, "Speed"=0.0}, {"Target Load"=0.0, "Target Disp"=0.0, "Rate"=0.0, "Speed"=0.0}, {"Target Load"=0.0, "Target Disp"=0.0, "Rate"=0.0, "Speed"=0.0}, {"Target Load"=0.0, "Target Disp"=0.0, "Rate"=0.0, "Speed"=0.0}, {"Target Load"=0.0, "Target Disp"=0.0, "Rate"=0.0, "Speed"=0.0}, {"Target Load"=0.0, "Target Disp"=0.0, "Rate"=0.0, "Speed"=0.0}, {"Target Load"=0.0, "Target Disp"=0.0, "Rate"=0.0, "Speed"=0.0}, {"Target Load"=0.0, "Target Disp"=0.0, "Rate"=0.0, "Speed"=0.0}, {"Target Load"=0.0, "Target Disp"=0.0, "Rate"=0.0, "Speed"=0.0}, {"Target Load"=0.0, "Target Disp"=0.0, "Rate"=0.0, "Speed"=0.0}, {"Target Load"=0.0, "Target Disp"=0.0, "Rate"=0.0, "Speed"=0.0}, {"Target Load"=0.0, "Target Disp"=0.0, "Rate"=0.0, "Speed"=0.0}, {"Target Load"=0.0, "Target Disp"=0.0, "Rate"=0.0, "Speed"=0.0}] ("Test")) -> ()
      n341 = global write "Global - System.vi" "System"(T24 [{"Out Type"=0, "Inverse"=0, "Monitor"=0, "Reserve"=0, "ACC Time"=0, "Pulse Rev"=0, "Stroke"=0, "Auto Off"=0, "Gear Ratio"=0.0, "Pitch"=0.0, "Max Speed"=0, "Jog Speed"=0, "Disp Coff"=0.0, "Max Load"=0}, {"Out Type"=0, "Inverse"=0, "Monitor"=0, "Reserve"=0, "ACC Time"=0, "Pulse Rev"=0, "Stroke"=0, "Auto Off"=0, "Gear Ratio"=0.0, "Pitch"=0.0, "Max Speed"=0, "Jog Speed"=0, "Disp Coff"=0.0, "Max Load"=0}, {"Out Type"=0, "Inverse"=0, "Monitor"=0, "Reserve"=0, "ACC Time"=0, "Pulse Rev"=0, "Stroke"=0, "Auto Off"=0, "Gear Ratio"=0.0, "Pitch"=0.0, "Max Speed"=0, "Jog Speed"=0, "Disp Coff"=0.0, "Max Load"=0}, {"Out Type"=0, "Inverse"=0, "Monitor"=0, "Reserve"=0, "ACC Time"=0, "Pulse Rev"=0, "Stroke"=0, "Auto Off"=0, "Gear Ratio"=0.0, "Pitch"=0.0, "Max Speed"=0, "Jog Speed"=0, "Disp Coff"=0.0, "Max Load"=0}, {"Out Type"=0, "Inverse"=0, "Monitor"=0, "Reserve"=0, "ACC Time"=0, "Pulse Rev"=0, "Stroke"=0, "Auto Off"=0, "Gear Ratio"=0.0, "Pitch"=0.0, "Max Speed"=0, "Jog Speed"=0, "Disp Coff"=0.0, "Max Load"=0}, {"Out Type"=0, "Inverse"=0, "Monitor"=0, "Reserve"=0, "ACC Time"=0, "Pulse Rev"=0, "Stroke"=0, "Auto Off"=0, "Gear Ratio"=0.0, "Pitch"=0.0, "Max Speed"=0, "Jog Speed"=0, "Disp Coff"=0.0, "Max Load"=0}, {"Out Type"=0, "Inverse"=0, "Monitor"=0, "Reserve"=0, "ACC Time"=0, "Pulse Rev"=0, "Stroke"=0, "Auto Off"=0, "Gear Ratio"=0.0, "Pitch"=0.0, "Max Speed"=0, "Jog Speed"=0, "Disp Coff"=0.0, "Max Load"=0}, {"Out Type"=0, "Inverse"=0, "Monitor"=0, "Reserve"=0, "ACC Time"=0, "Pulse Rev"=0, "Stroke"=0, "Auto Off"=0, "Gear Ratio"=0.0, "Pitch"=0.0, "Max Speed"=0, "Jog Speed"=0, "Disp Coff"=0.0, "Max Load"=0}, {"Out Type"=0, "Inverse"=0, "Monitor"=0, "Reserve"=0, "ACC Time"=0, "Pulse Rev"=0, "Stroke"=0, "Auto Off"=0, "Gear Ratio"=0.0, "Pitch"=0.0, "Max Speed"=0, "Jog Speed"=0, "Disp Coff"=0.0, "Max Load"=0}, {"Out Type"=0, "Inverse"=0, "Monitor"=0, "Reserve"=0, "ACC Time"=0, "Pulse Rev"=0, "Stroke"=0, "Auto Off"=0, "Gear Ratio"=0.0, "Pitch"=0.0, "Max Speed"=0, "Jog Speed"=0, "Disp Coff"=0.0, "Max Load"=0}, {"Out Type"=0, "Inverse"=0, "Monitor"=0, "Reserve"=0, "ACC Time"=0, "Pulse Rev"=0, "Stroke"=0, "Auto Off"=0, "Gear Ratio"=0.0, "Pitch"=0.0, "Max Speed"=0, "Jog Speed"=0, "Disp Coff"=0.0, "Max Load"=0}, {"Out Type"=0, "Inverse"=0, "Monitor"=0, "Reserve"=0, "ACC Time"=0, "Pulse Rev"=0, "Stroke"=0, "Auto Off"=0, "Gear Ratio"=0.0, "Pitch"=0.0, "Max Speed"=0, "Jog Speed"=0, "Disp Coff"=0.0, "Max Load"=0}, {"Out Type"=0, "Inverse"=0, "Monitor"=0, "Reserve"=0, "ACC Time"=0, "Pulse Rev"=0, "Stroke"=0, "Auto Off"=0, "Gear Ratio"=0.0, "Pitch"=0.0, "Max Speed"=0, "Jog Speed"=0, "Disp Coff"=0.0, "Max Load"=0}, {"Out Type"=0, "Inverse"=0, "Monitor"=0, "Reserve"=0, "ACC Time"=0, "Pulse Rev"=0, "Stroke"=0, "Auto Off"=0, "Gear Ratio"=0.0, "Pitch"=0.0, "Max Speed"=0, "Jog Speed"=0, "Disp Coff"=0.0, "Max Load"=0}, {"Out Type"=0, "Inverse"=0, "Monitor"=0, "Reserve"=0, "ACC Time"=0, "Pulse Rev"=0, "Stroke"=0, "Auto Off"=0, "Gear Ratio"=0.0, "Pitch"=0.0, "Max Speed"=0, "Jog Speed"=0, "Disp Coff"=0.0, "Max Load"=0}, {"Out Type"=0, "Inverse"=0, "Monitor"=0, "Reserve"=0, "ACC Time"=0, "Pulse Rev"=0, "Stroke"=0, "Auto Off"=0, "Gear Ratio"=0.0, "Pitch"=0.0, "Max Speed"=0, "Jog Speed"=0, "Disp Coff"=0.0, "Max Load"=0}] ("System")) -> ()
      n342 = global write "Global - IP Address.vi" "IP"(w902) -> ()
      n343 = global write "Global - Unit.vi" "Unit"(T27 [{"Name"=[], "Unit"=[], "Decimal Point"=[], "Ch Log"=[], "H Alarm"=[], "L Alarm"=[], "H Limit"=[], "L Limit"=[], "Filter"=[], "Gain"=[], "Calib Type"=[]}, {"Name"=[], "Unit"=[], "Decimal Point"=[], "Ch Log"=[], "H Alarm"=[], "L Alarm"=[], "H Limit"=[], "L Limit"=[], "Filter"=[], "Gain"=[], "Calib Type"=[]}, {"Name"=[], "Unit"=[], "Decimal Point"=[], "Ch Log"=[], "H Alarm"=[], "L Alarm"=[], "H Limit"=[], "L Limit"=[], "Filter"=[], "Gain"=[], "Calib Type"=[]}, {"Name"=[], "Unit"=[], "Decimal Point"=[], "Ch Log"=[], "H Alarm"=[], "L Alarm"=[], "H Limit"=[], "L Limit"=[], "Filter"=[], "Gain"=[], "Calib Type"=[]}, {"Name"=[], "Unit"=[], "Decimal Point"=[], "Ch Log"=[], "H Alarm"=[], "L Alarm"=[], "H Limit"=[], "L Limit"=[], "Filter"=[], "Gain"=[], "Calib Type"=[]}, {"Name"=[], "Unit"=[], "Decimal Point"=[], "Ch Log"=[], "H Alarm"=[], "L Alarm"=[], "H Limit"=[], "L Limit"=[], "Filter"=[], "Gain"=[], "Calib Type"=[]}, {"Name"=[], "Unit"=[], "Decimal Point"=[], "Ch Log"=[], "H Alarm"=[], "L Alarm"=[], "H Limit"=[], "L Limit"=[], "Filter"=[], "Gain"=[], "Calib Type"=[]}, {"Name"=[], "Unit"=[], "Decimal Point"=[], "Ch Log"=[], "H Alarm"=[], "L Alarm"=[], "H Limit"=[], "L Limit"=[], "Filter"=[], "Gain"=[], "Calib Type"=[]}, {"Name"=[], "Unit"=[], "Decimal Point"=[], "Ch Log"=[], "H Alarm"=[], "L Alarm"=[], "H Limit"=[], "L Limit"=[], "Filter"=[], "Gain"=[], "Calib Type"=[]}, {"Name"=[], "Unit"=[], "Decimal Point"=[], "Ch Log"=[], "H Alarm"=[], "L Alarm"=[], "H Limit"=[], "L Limit"=[], "Filter"=[], "Gain"=[], "Calib Type"=[]}, {"Name"=[], "Unit"=[], "Decimal Point"=[], "Ch Log"=[], "H Alarm"=[], "L Alarm"=[], "H Limit"=[], "L Limit"=[], "Filter"=[], "Gain"=[], "Calib Type"=[]}, {"Name"=[], "Unit"=[], "Decimal Point"=[], "Ch Log"=[], "H Alarm"=[], "L Alarm"=[], "H Limit"=[], "L Limit"=[], "Filter"=[], "Gain"=[], "Calib Type"=[]}, {"Name"=[], "Unit"=[], "Decimal Point"=[], "Ch Log"=[], "H Alarm"=[], "L Alarm"=[], "H Limit"=[], "L Limit"=[], "Filter"=[], "Gain"=[], "Calib Type"=[]}, {"Name"=[], "Unit"=[], "Decimal Point"=[], "Ch Log"=[], "H Alarm"=[], "L Alarm"=[], "H Limit"=[], "L Limit"=[], "Filter"=[], "Gain"=[], "Calib Type"=[]}, {"Name"=[], "Unit"=[], "Decimal Point"=[], "Ch Log"=[], "H Alarm"=[], "L Alarm"=[], "H Limit"=[], "L Limit"=[], "Filter"=[], "Gain"=[], "Calib Type"=[]}, {"Name"=[], "Unit"=[], "Decimal Point"=[], "Ch Log"=[], "H Alarm"=[], "L Alarm"=[], "H Limit"=[], "L Limit"=[], "Filter"=[], "Gain"=[], "Calib Type"=[]}] ("Unit")) -> ()
      n344 = global write "Global - ADC.vi" "ADC"(T26 [{"Active Ch"=[], "Filter Type"=0, "Post Filter"=[], "Gain"=[], "FS"=0, "IntOC"=0, "IntFC"=0, "SysOC"=0, "Cofficient"=[], "K"=[], "Max"=0}, {"Active Ch"=[], "Filter Type"=0, "Post Filter"=[], "Gain"=[], "FS"=0, "IntOC"=0, "IntFC"=0, "SysOC"=0, "Cofficient"=[], "K"=[], "Max"=0}, {"Active Ch"=[], "Filter Type"=0, "Post Filter"=[], "Gain"=[], "FS"=0, "IntOC"=0, "IntFC"=0, "SysOC"=0, "Cofficient"=[], "K"=[], "Max"=0}, {"Active Ch"=[], "Filter Type"=0, "Post Filter"=[], "Gain"=[], "FS"=0, "IntOC"=0, "IntFC"=0, "SysOC"=0, "Cofficient"=[], "K"=[], "Max"=0}, {"Active Ch"=[], "Filter Type"=0, "Post Filter"=[], "Gain"=[], "FS"=0, "IntOC"=0, "IntFC"=0, "SysOC"=0, "Cofficient"=[], "K"=[], "Max"=0}, {"Active Ch"=[], "Filter Type"=0, "Post Filter"=[], "Gain"=[], "FS"=0, "IntOC"=0, "IntFC"=0, "SysOC"=0, "Cofficient"=[], "K"=[], "Max"=0}, {"Active Ch"=[], "Filter Type"=0, "Post Filter"=[], "Gain"=[], "FS"=0, "IntOC"=0, "IntFC"=0, "SysOC"=0, "Cofficient"=[], "K"=[], "Max"=0}, {"Active Ch"=[], "Filter Type"=0, "Post Filter"=[], "Gain"=[], "FS"=0, "IntOC"=0, "IntFC"=0, "SysOC"=0, "Cofficient"=[], "K"=[], "Max"=0}, {"Active Ch"=[], "Filter Type"=0, "Post Filter"=[], "Gain"=[], "FS"=0, "IntOC"=0, "IntFC"=0, "SysOC"=0, "Cofficient"=[], "K"=[], "Max"=0}, {"Active Ch"=[], "Filter Type"=0, "Post Filter"=[], "Gain"=[], "FS"=0, "IntOC"=0, "IntFC"=0, "SysOC"=0, "Cofficient"=[], "K"=[], "Max"=0}, {"Active Ch"=[], "Filter Type"=0, "Post Filter"=[], "Gain"=[], "FS"=0, "IntOC"=0, "IntFC"=0, "SysOC"=0, "Cofficient"=[], "K"=[], "Max"=0}, {"Active Ch"=[], "Filter Type"=0, "Post Filter"=[], "Gain"=[], "FS"=0, "IntOC"=0, "IntFC"=0, "SysOC"=0, "Cofficient"=[], "K"=[], "Max"=0}, {"Active Ch"=[], "Filter Type"=0, "Post Filter"=[], "Gain"=[], "FS"=0, "IntOC"=0, "IntFC"=0, "SysOC"=0, "Cofficient"=[], "K"=[], "Max"=0}, {"Active Ch"=[], "Filter Type"=0, "Post Filter"=[], "Gain"=[], "FS"=0, "IntOC"=0, "IntFC"=0, "SysOC"=0, "Cofficient"=[], "K"=[], "Max"=0}, {"Active Ch"=[], "Filter Type"=0, "Post Filter"=[], "Gain"=[], "FS"=0, "IntOC"=0, "IntFC"=0, "SysOC"=0, "Cofficient"=[], "K"=[], "Max"=0}, {"Active Ch"=[], "Filter Type"=0, "Post Filter"=[], "Gain"=[], "FS"=0, "IntOC"=0, "IntFC"=0, "SysOC"=0, "Cofficient"=[], "K"=[], "Max"=0}] ("ADC")) -> ()
      n345 = global write "Global - Comport.vi" "Port"(string[] [] ("Comport")) -> ()
    }
    frame Error {
    }
  }
